vi "Facade.vi"(0 "Data In":T6, 2 "Display State In":T3, 3 "Container State":T5) -> (6 "Data Out":T6, 7 "Display State Out":T3, 8 "Action":T2)   [LabVIEW 2017, in "3D Mesh.xctl"]
uses:
  <vilib>/Math Plots/3D Math Plots/3D Mesh/3D Mesh XCtrl/3D Mesh.xctl
  <vilib>/Math Plots/3D Math Plots/3D Mesh/3D Mesh XCtrl/Data.ctl
  <vilib>/Math Plots/3D Math Plots/3D Plot/3D Plot Datatype/3D Plot Datatype.lvclass
  <vilib>/_xctls/Container State.ctl
  <vilib>/Math Plots/3D Math Plots/3D Mesh/3D Mesh XCtrl/State.ctl
  <vilib>/Math Plots/3D Math Plots/3D Mesh/3D Mesh/3D Mesh.lvclass
  e:/builds/penguin/labview/branches/2017/dev/dist/vi.lib/Math Plots/3D Math Plots/3D Plot/3D Plot/3D Plot.lvclass
  <vilib>/Math Plots/3D Math Plots/3D Plot/Action String/3DMathPlot Ctrl Act Queue.ctl
  <vilib>/Math Plots/3D Math Plots/3D Plot/Action String/3DMathPlot Ctrl Act Cluster.ctl
  <vilib>/Math Plots/3D Math Plots/3D Plot/Action String/3DMathPlot State Class.ctl
  <vilib>/_xctls/Action.ctl
  <vilib>/Math Plots/3D Math Plots/3D Plot/3D Plot/Typedef/Plot Action.ctl
  <vilib>/Math Plots/3D Math Plots/3D Plot/Action String/3DMathPlot Action String.ctl
  <vilib>/_xctls/XControlSupport.lvlib
  <vilib>/Math Plots/3D Math Plots/3D Plot/3D Plot/3D Plot.lvclass
panel:
  out "Export Image":picture
  out "3D Picture Control":refnum<vi>(3d-picture)
  in  "XY Graph":cluster{dbl, dbl}[](graph)
  out "Render Window":refnum<vi>
  in  "Projection Palette":T1
  out "Intensity Graph":dbl[][](graph)
  in  "Color Ramp Palette":cluster{"Active Plot":i32} {"Active Plot" items=["Plot-1"]}
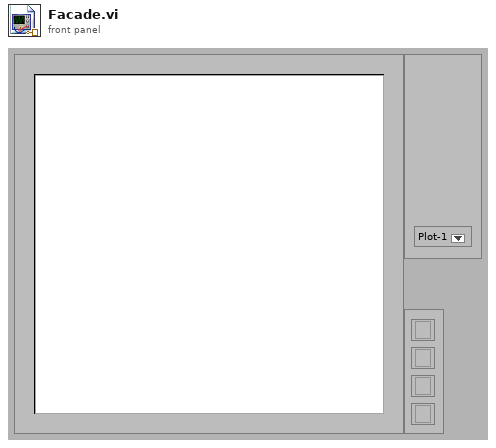
[diagram p1: front panel]
types:
  T1 = cluster{"XY Projection":bool, "XZ Projection":bool, "YZ Projection":bool, "3D Projection":bool}
  T2 = typedef "XControlSupport.lvlib/Action.ctl" = cluster{"Data Changed?":bool, "State Changed?":bool, "Action Name":string}
  T3 = typedef "3D Mesh.xctl/State.ctl" = cluster{"3D Mesh.lvclass":refnum<class "3D Mesh.lvclass">, "Control Ref Queue":T4, "Main Frame Color":u32, "Ramp Palette Color":u32, "Projection Palette Color":u32}
  T4 = typedef "3DMathPlot Ctrl Act Queue.ctl" = refnum<queue>
  T5 = typedef "XControlSupport.lvlib/Container State.ctl" = cluster{"Indicator?":bool, "Run Mode?":bool, " Refnum":refnum<vi>}
  T6 = typedef "3D Mesh.xctl/Data.ctl" = refnum<class "3D Plot Datatype.lvclass">[]
  T7 = typedef "3DMathPlot Ctrl Act Cluster.ctl" = cluster{"3D Picture Control":refnum<vi>, "Render Window Refnum":refnum<vi>, "XY Graph":refnum<vi>, "Intensity Graph":refnum<vi>, "Color Legend Palette":refnum<vi>, "Projection Palette":refnum<vi>, "XControl  Ref":refnum<vi>, "Facade Ref":refnum<vi>, "Export Image Ref":refnum<vi>, "Clear Data Flag":bool, "Display State Change Class":T8}
  T8 = typedef "3DMathPlot State Class.ctl" = enum16{"Update All Objects (Undo)", "Update Light Object Only", "Update Axis Object Only", "Update Plot Object Only", "Update Cursor Object Only", "Update Axis Plot Cursor Objects", "No Update"}
  T9 = typedef "3D Plot.lvclass/Plot Action.ctl" = cluster{"Light Action":enum16{"Update", "Remove", "Nothing"}, "Axis Action":enum16{"Update", "Remove", "Nothing"}, "Plot Action":enum16{"Update", "Remove", "Nothing"}, "Cursor Action":enum16{"Update", "Remove", "Nothing"}, "Fast Draw Action":enum16{"Update", "Remove", "Nothing"}}
  T10 = enum32{"Towards X-Y Plane", "Towards X-Z Plane", "Towards Y-Z Plane", "User Defined"}
  T11 = typedef "3D Plot.lvclass/Actual Transform.ctl" = cluster{"Scale Cluster":cluster{"X Scale":sgl, "Y Scale":sgl, "Z Scale":sgl}, "Translate Cluster":cluster{"X Translate":sgl, "Y Translate":sgl, "Z Translate":sgl}, "Actual Range":T12}
  T12 = typedef "3D Plot.lvclass/Range Clusters.ctl" = cluster{"X Range":cluster{"Max X":sgl, "Min X":sgl}, "Y Range":cluster{"Max Y":sgl, "Min Y":sgl}, "Z Range":cluster{"Max Z":sgl, "Min Z":sgl}}
  T13 = typedef "3D Plot.lvclass/Multiplot Representation.ctl" = cluster{"Plot Represention Array":T14[], "Max Range":T12}
  T14 = typedef "3D Plot.lvclass/Plot Representation.ctl" = cluster{"Plot ID":i32, "Plot Range":T12, "Mesh Data":T15, "Dimension":cluster{"X Dimension":i32, "Y Dimension":i32}, "Ramp Range":T12}
  T15 = typedef "3D Plot.lvclass/Mesh Data.ctl" = cluster{"Index Array":u32[], "Vertex Array":cluster{"X":sgl, "Y":sgl, "Z":sgl}[], "Normal Array":cluster{"X":sgl, "Y":sgl, "Z":sgl}[], "Color Index Array":i32[]}
  T16 = typedef "3D Plot.lvclass/Object Cluster.ctl" = cluster{"Root Scene Object":refnum<vi>, "Fast Root Scene Object":refnum<vi>}
  T17 = typedef "3DMathPlot Action String.ctl" = u16
  T18 = typedef "3D Plot.lvclass/Property Cluster.ctl" = cluster{"Graph Property":T19, "Light Property":T23, "Axis Property":T25, "Value Pair Property":T31, "Format Property":T33, "Cursor Property Array":T34, "Appearance Property":T43}
  T19 = typedef "3D Plot.lvclass/Graph Property.ctl" = cluster{"General Property":T20, "View Property":T21, "Grid Plane":T22}
  T20 = typedef "3D Plot.lvclass/General Property.ctl" = cluster{"Plot Area Color":u32, "Fast Draw?":bool, "Clip Data?":bool}
  T21 = typedef "3D Plot.lvclass/View Property.ctl" = cluster{"Projection Mode":enum16{"Orthographic", "Perspective"}, "View Direction":enum32{"Towards X-Y Plane", "Towards X-Z Plane", "Towards Y-Z Plane", "User Defined"}, "User Defined View Direction":cluster{"View Latitude":sgl, "View Longitude":sgl, "View Distance":sgl}}
  T22 = typedef "3D Plot.lvclass/Grid Plane.ctl" = cluster{"Grid Plane Visible":cluster{"Draw Grid Plane X-Y":bool, "Draw Grid Plane Y-Z":bool, "Draw Grid Plane X-Z":bool}, "Grid Antialiasing":bool, "Grid Frame Color":u32}
  T23 = typedef "3D Plot.lvclass/Light Property.ctl" = cluster{"Enable Lighting?":bool, "Ambient Color":u32, "Light Array":T24[]}
  T24 = typedef "3D Plot.lvclass/Light Specific.ctl" = cluster{"Enable Light?":bool, "Light Color":u32, "Light Latitude":sgl, "Light Longitude":sgl, "Light Distance":sgl, "Attenuation":enum16{"None", "Linear", "Quadratic"}}
  T25 = typedef "3D Plot.lvclass/Axis Property.ctl" = cluster{"Caption Property":T26, "Label Property":T27, "Range Property":T28, "Grid Property":T29, "Ticks Property":T30}
  T26 = typedef "3D Plot.lvclass/Caption Property.ctl" = cluster{"Show Caption":cluster{"Show Normal X Caption":bool, "Show Normal Y Caption":bool, "Show Normal Z Caption":bool, "Show Opposite X Caption":bool, "Show Opposite Y Caption":bool, "Show Opposite Z Caption":bool}, "Caption Color":cluster{"Caption Color X":u32, "Caption Color Y":u32, "Caption Color Z":u32}, "Caption Size":cluster{"Caption Size X":u16, "Caption Size Y":u16, "Caption Size Z":u16}, "Caption String":cluster{"Caption X":string, "Caption Y":string, "Caption Z ":string}}
  T27 = typedef "3D Plot.lvclass/Label Property.ctl" = cluster{"Show Label":cluster{"Show Normal X Label":bool, "Show Normal Y Label":bool, "Show Normal Z Label":bool, "Show Opposite X Label":bool, "Show Opposite Y Label":bool, "Show Opposite Z Label":bool}, "Label Color":cluster{"Label Color X":u32, "Label Color Y":u32, "Label Color Z":u32}, "Label Size":cluster{"Label Size X":u16, "Label Size Y":u16, "Labe Size Z":u16}}
  T28 = typedef "3D Plot.lvclass/Range Property.ctl" = cluster{"Range Cluster":T12, "Auto Range":cluster{"Auto Range X":bool, "Auto Range Y":bool, "Auto Range Z":bool}, "Inverted":cluster{"Inverted X":bool, "Inverted Y":bool, "Inverted Z":bool}, "Logarithm":cluster{"Logarithm X":bool, "Logarithm Y":bool, "Logarithm Z":bool}}
  T29 = typedef "3D Plot.lvclass/Grid Property.ctl" = cluster{"Major Grid Visible":cluster{"Draw Major Grid X":bool, "Draw Major Grid Y":bool, "Draw Major Grid Z":bool}, "Major Grid Color":cluster{"Major Grid Color X":u32, "Major Grid Color Y":u32, "Major Grid Color Z":u32}, "Minor Grid Visible":cluster{"Draw Minor Grid X":bool, "Draw Minor Grid Y":bool, "Draw Minor Grid Z":bool}, "Minor Grid Color":cluster{"Minor Grid Color X":u32, "Minor Grid Color Y":u32, "Minor Grid Color Z":u32}}
  T30 = typedef "3D Plot.lvclass/Tick Property.ctl" = cluster{"Major Tick Visible":cluster{"Draw Major Tick X":bool, "Draw Major Tick Y":bool, "Draw Major Tick Z":bool}, "Major Tick Color":cluster{"Major Tick Color X":u32, "Major Tick Color Y":u32, "Major Tick Color Z":u32}, "Major Count":cluster{"Major Count X":u16, "Major Count Y":u16, "Major Count Z":u16}, "Minor Tick Visible":cluster{"Draw Minor Tick X":bool, "Draw Minor Tick Y":bool, "Draw Minor Tick Z":bool}, "Minor Tick Color":cluster{"Minor Tick Color X":u32, "Minor Tick Color Y":u32, "Minor Tick Color Z":u32}, "Minor Count":cluster{"Minor Count X":u16, "Minor Count Y":u16, "Minor Count Z":u16}}
  T31 = typedef "3D Plot.lvclass/Value Pair Property.ctl" = T32[]
  T32 = typedef "3D Plot.lvclass/Value Pair Cluster.ctl" = cluster{"Value Pair Array":cluster{"Value":sgl, "Name":string}[], "Show Tick":bool, "Show Grid":bool, " Label Mode":enum16{"Name", "Value", "None"}}
  T33 = typedef "3D Plot.lvclass/Format Property.ctl" = string[]
  T34 = typedef "3D Plot.lvclass/Cursor Property Array.ctl" = T35[]
  T35 = typedef "3D Plot.lvclass/Cursor Property.ctl" = cluster{"Cursor Visible":bool, "Cursor Enable":bool, "Cursor Position":T36, "Cursor Point":T37, "Cursor Line":T39, "Cursor Plane":T41, "Cursor Text":T42}
  T36 = typedef "3D Plot.lvclass/Cursor Position.ctl" = cluster{"Cursor Plot ID":i32, "Cursor X":sgl, "Cursor Y":sgl, "Cursor Z":sgl, "Cursor Snap To":enum16{"Fixed", "Nearest Plot", "Snap to Plot"}}
  T37 = typedef "3D Plot.lvclass/Cursor Point.ctl" = cluster{"Cursor Point Color":u32, "Cursor Point Size":sgl, "Cursor Point Style":T38}
  T38 = typedef "3D Plot.lvclass/Sprite Type.ctl" = enum16{"None", "Empty Square", "Solid Square", "Empty Diamond", "Solid Diamond", "Empty Circle", "Solid Circle", "Asterisk", "Bold X", "Wireframe Sphere", "Solid Sphere", "Wireframe Cube", "Solid Cube"}
  T39 = typedef "3D Plot.lvclass/Cursor Line.ctl" = cluster{"Cursor Line Color":u32, "Cursor Line Width":sgl, "Cursor Line Style":T40}
  T40 = typedef "3D Plot.lvclass/Line Type.ctl" = enum16{"None", "Solid", "Dash", "Dot", "Dash Dot"}
  T41 = typedef "3D Plot.lvclass/Cursor Plane.ctl" = cluster{"Cursor Plane Color":u32, "Cursor Plane Opacity":sgl, "Draw Cursor Plane X-Z":bool, "Draw Cursor Plane Y-Z":bool, "Draw Cursor Plane X-Y":bool}
  T42 = typedef "3D Plot.lvclass/Cursor Text.ctl" = cluster{"Cursor Text":string, "Cursor Text Size":u16, "Cursor Show Position":bool, "Cursor Show Name":bool, "Cursor Text Color":u32, "Background Color":u32, "Background Opacity":sgl}
  T43 = typedef "3D Plot.lvclass/Apearance Property.ctl" = cluster{"Visibility":T44, "Active Index":cluster{"Active Plot":i32, "Active Cursor":i32, "Active Axis":enum16{"X-axis", "Y-axis", "Z-axis"}, "Active Value Pair":enum16{"X-axis", "Y-axis", "Z-axis"}, "Active Light":enum16{"Light 0", "Light 1", "Light 2", "Light 3"}}, "Backup Data":cluster{"Plot Name":string[]}}
  T44 = typedef "3D Plot.lvclass/Item Visibility.ctl" = cluster{"Projection Palette":bool, "Color Ramp Palette":bool}
  T45 = typedef "LVPoint32TypeDef.ctl" = cluster{"Horizontal":i32, "Vertical":i32}
  T46 = typedef "LVRangeTypeDef.ctl" = cluster{"Minimum":dbl, "Maximum":dbl, "Increment":dbl, "Minor Increment":dbl, "Start":dbl}
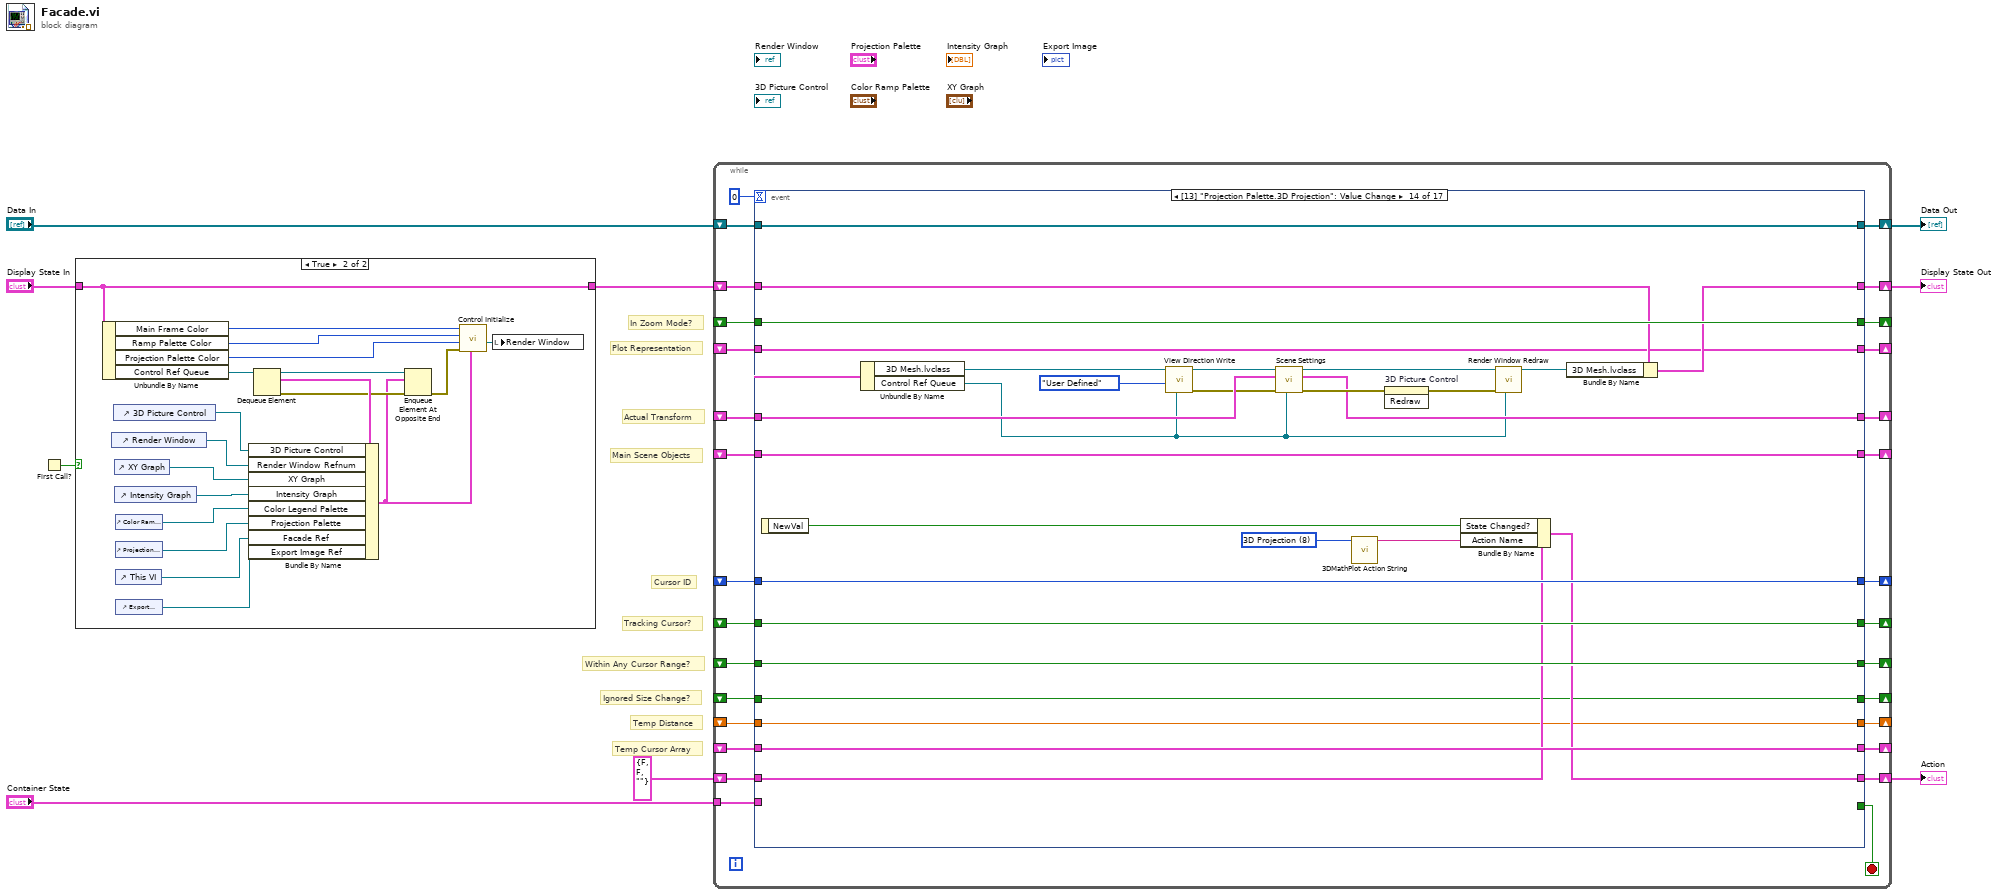
[diagram p0: block diagram]
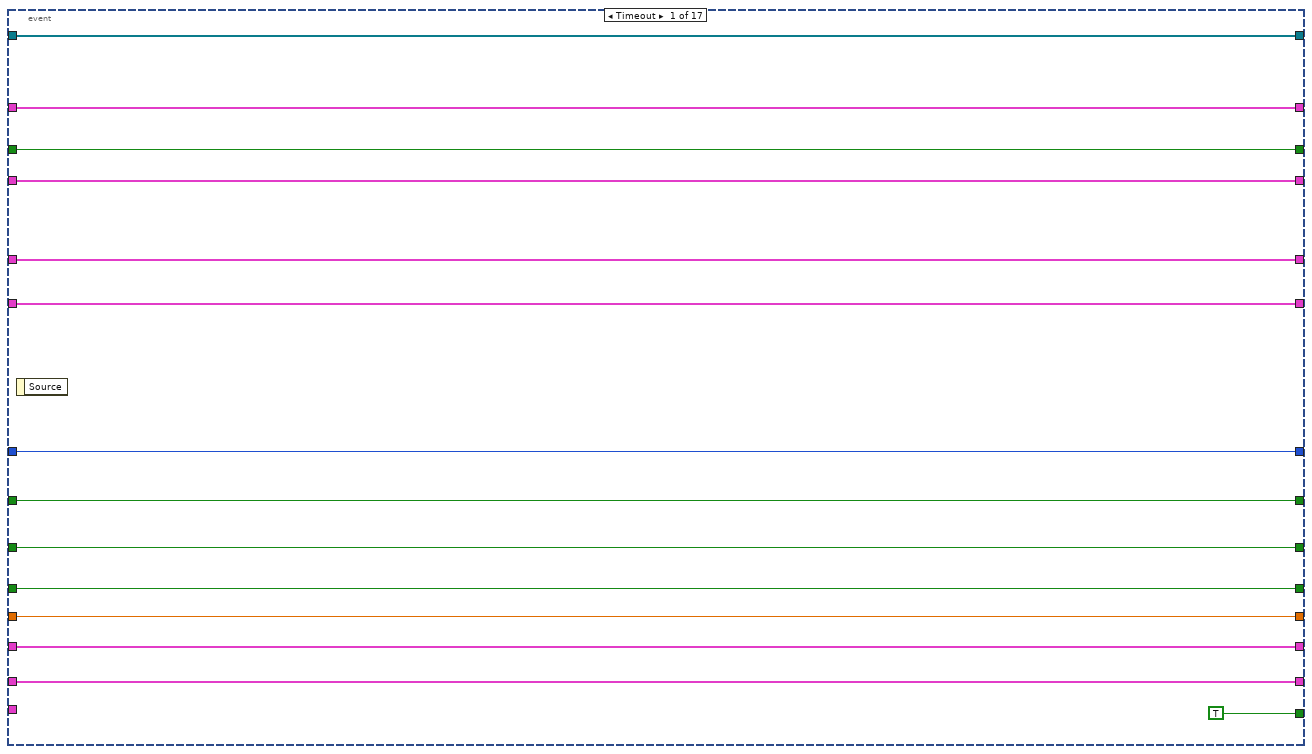
[diagram p3: hidden frame]
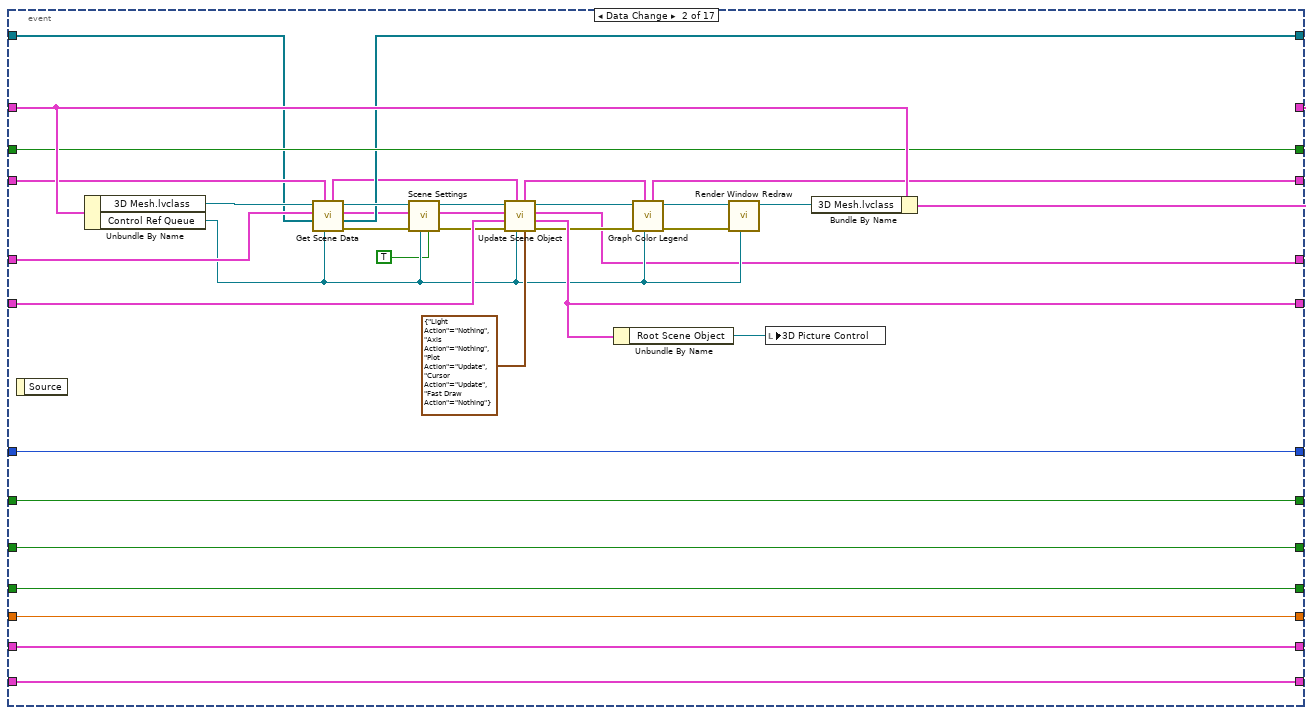
[diagram p4: hidden frame]
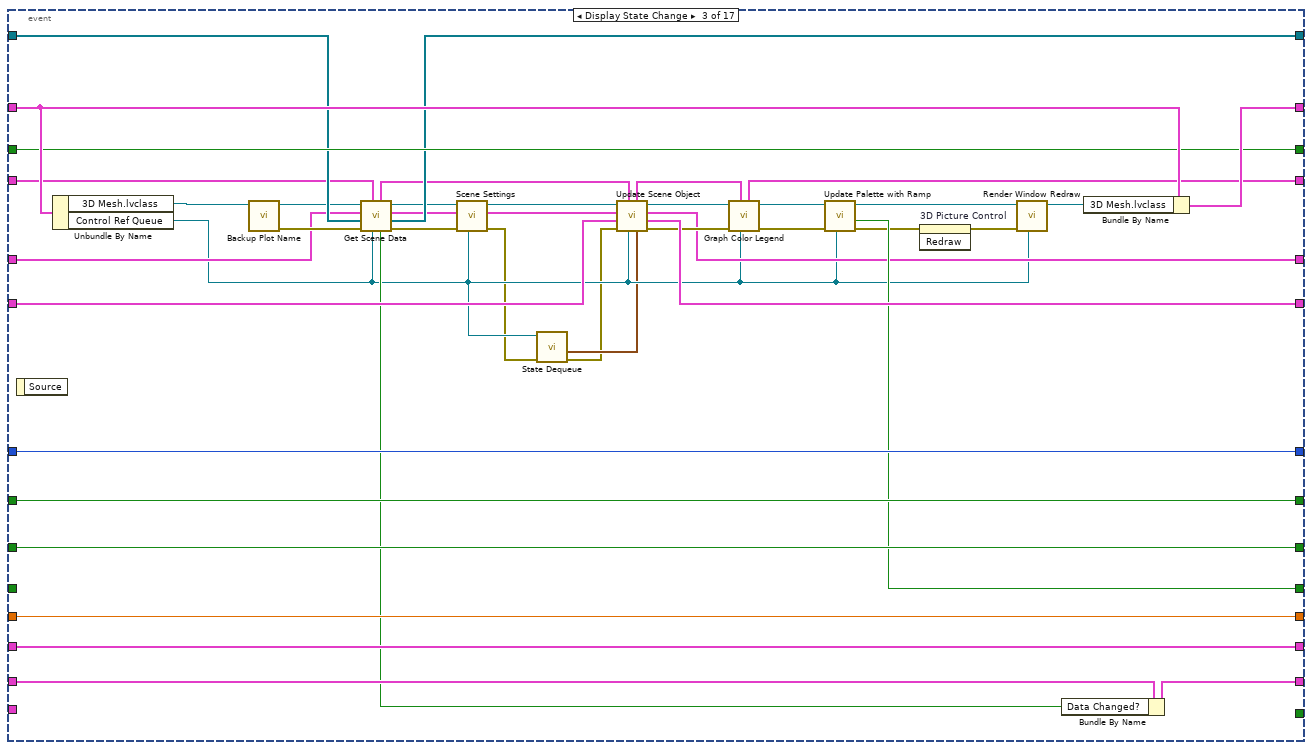
[diagram p5: hidden frame]
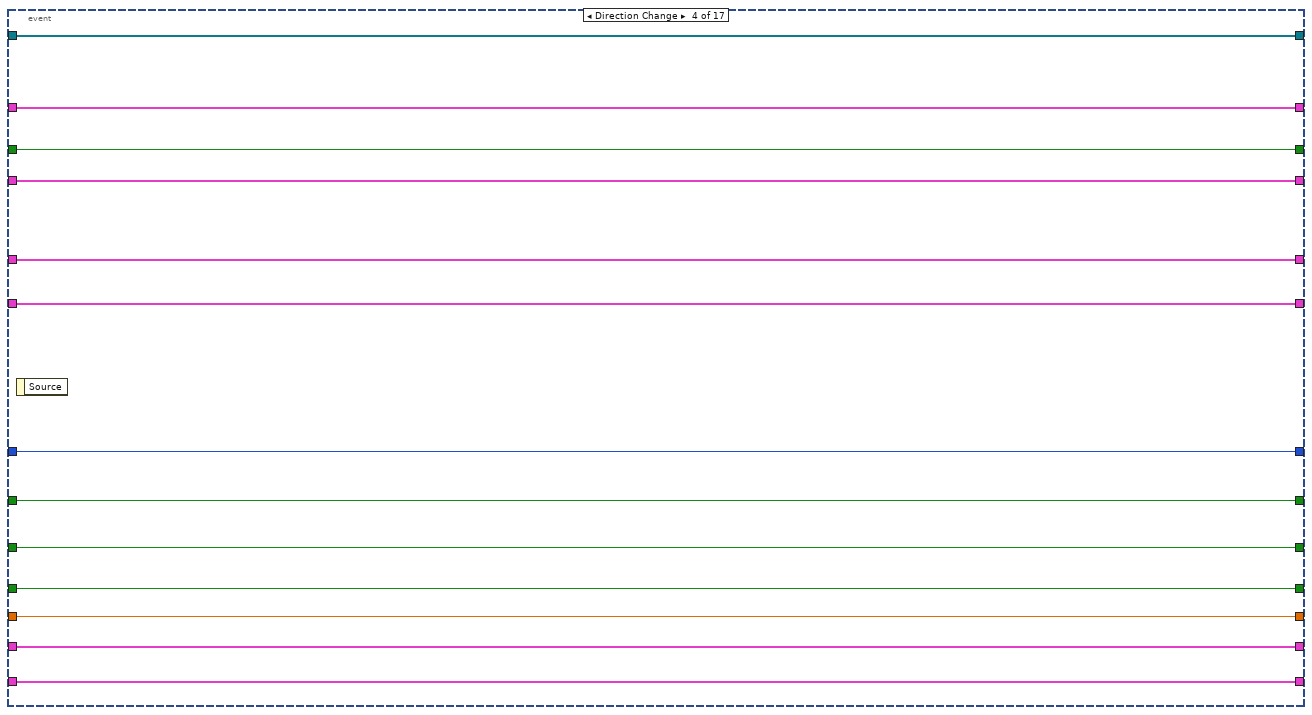
[diagram p6: hidden frame]
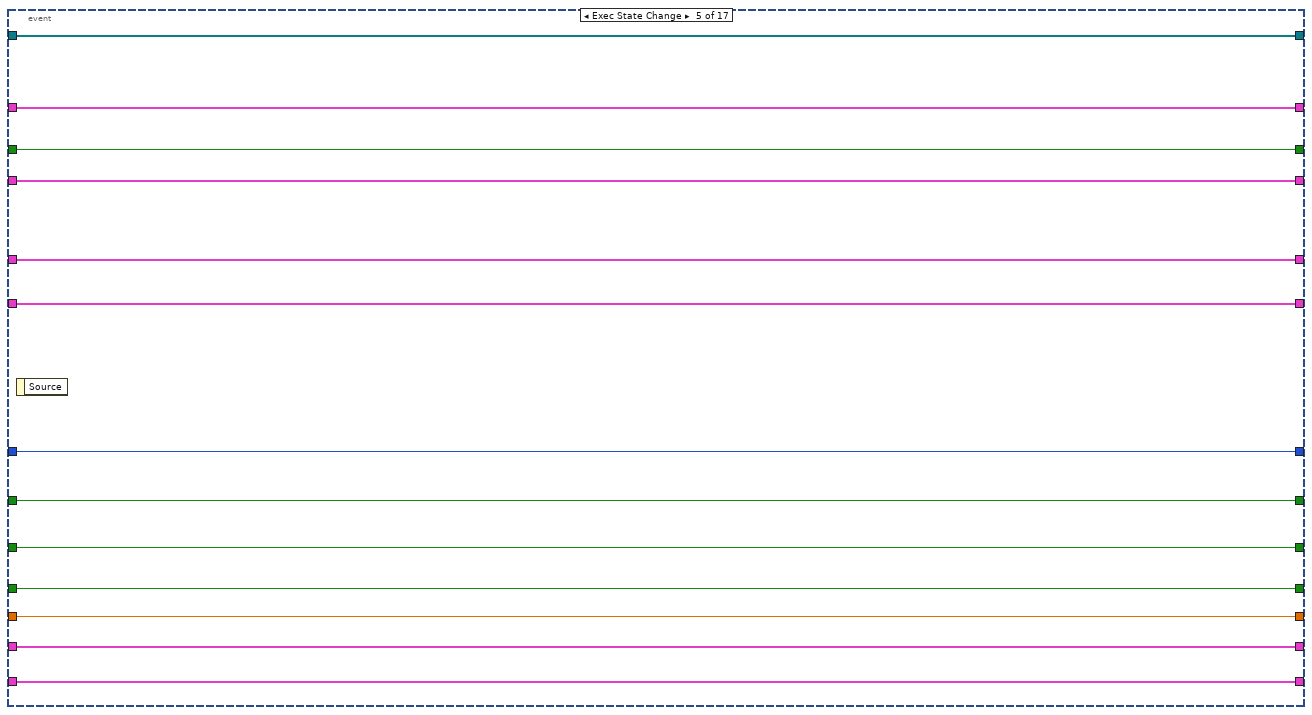
[diagram p7: hidden frame]
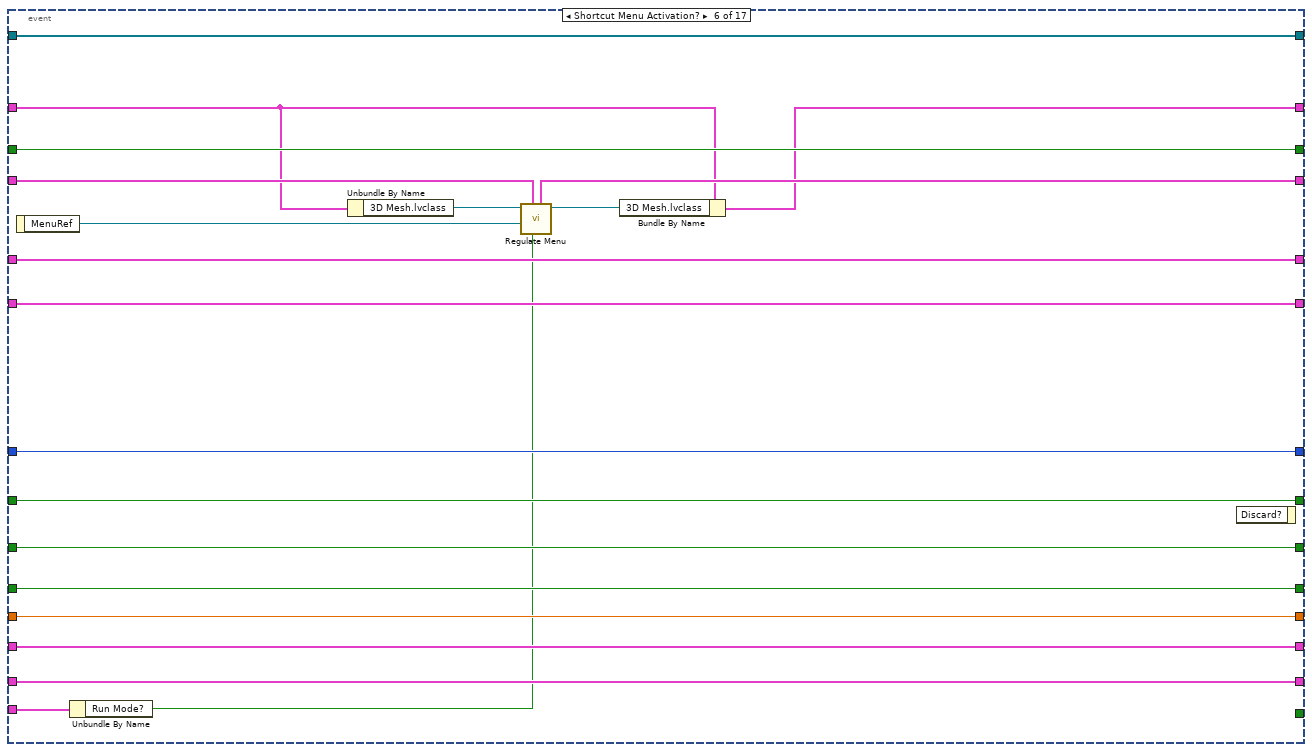
[diagram p8: hidden frame]
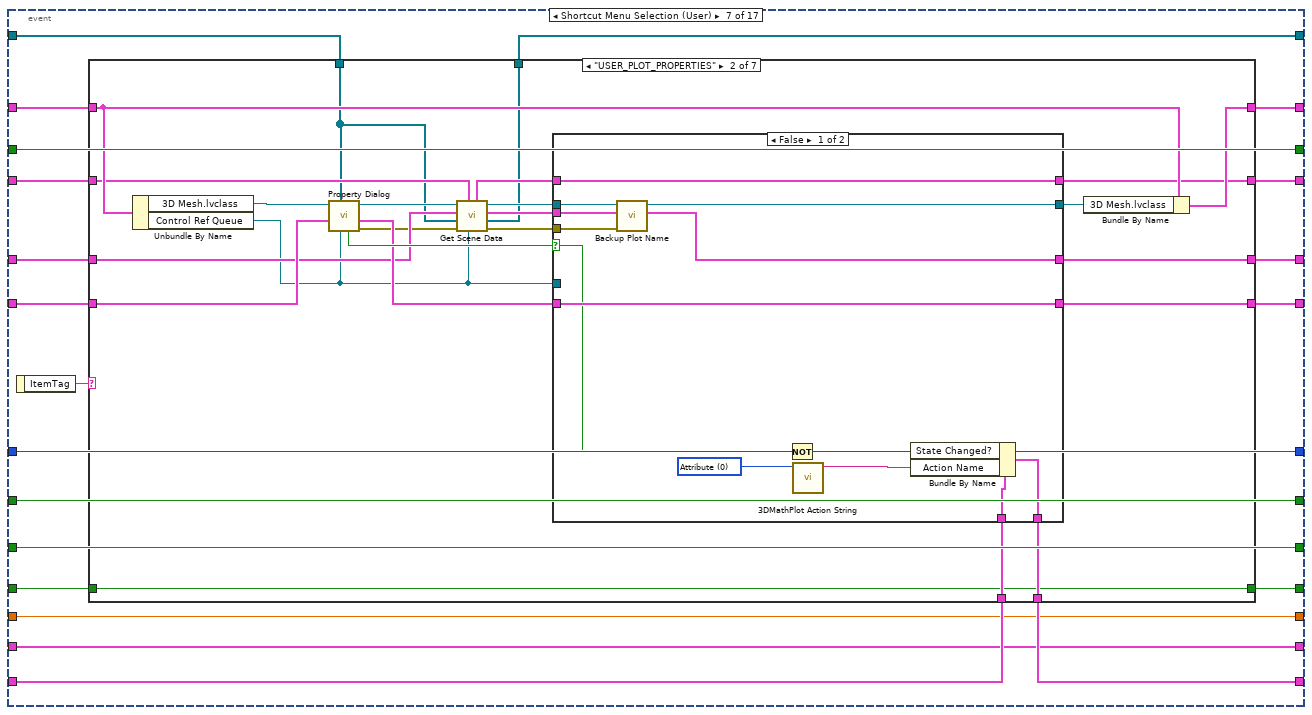
[diagram p9: hidden frame]
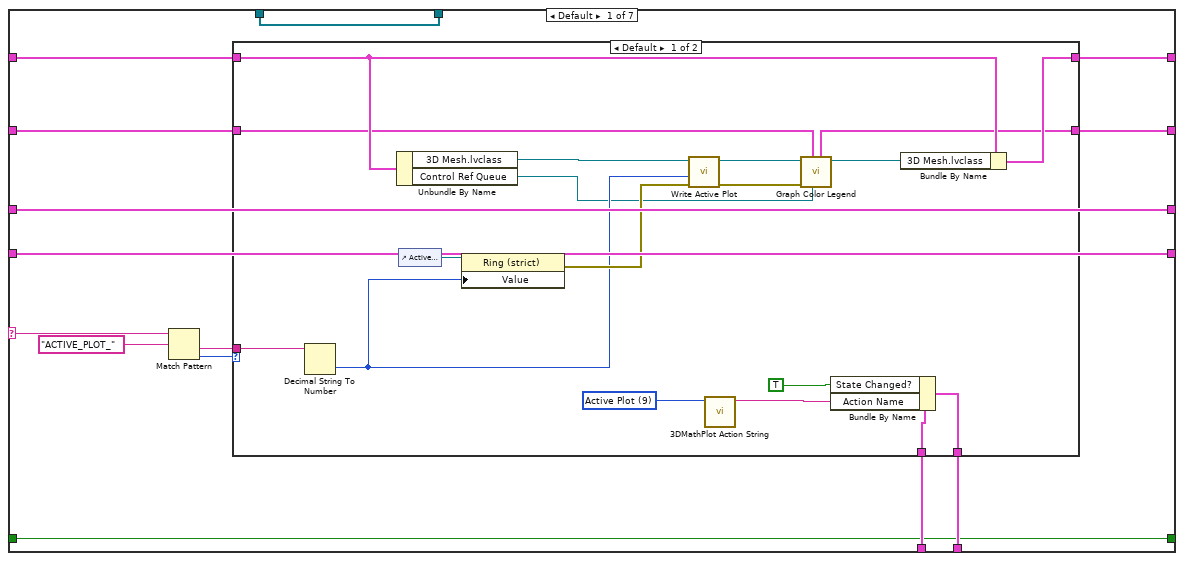
[diagram p10: hidden frame]
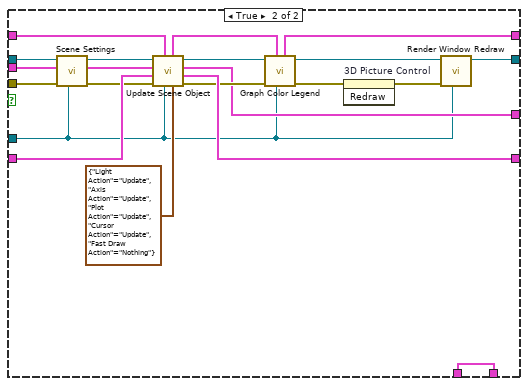
[diagram p12: hidden frame]
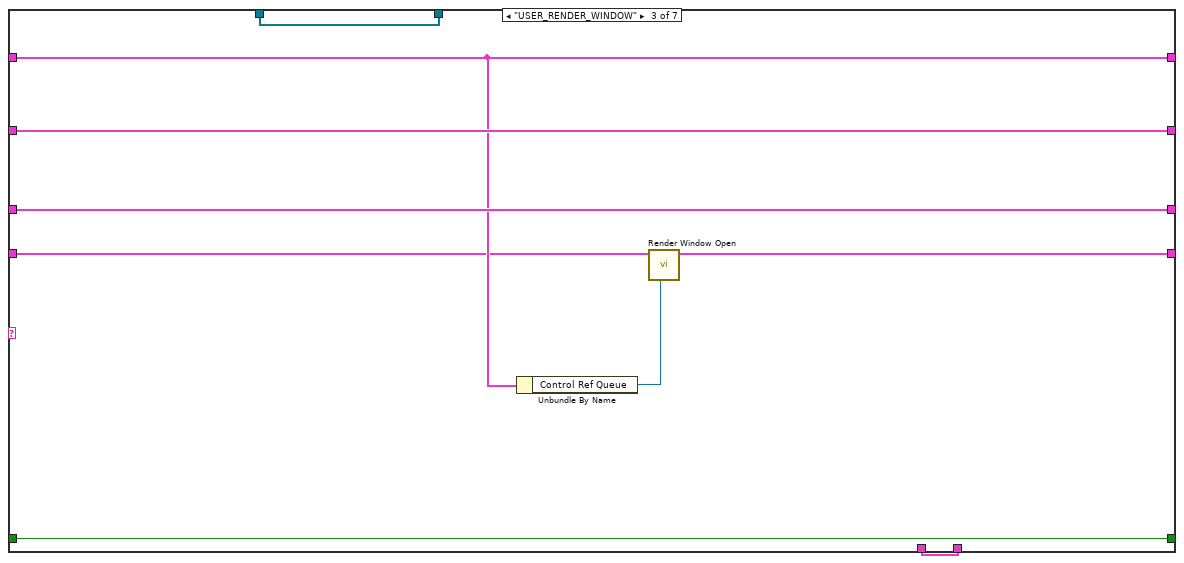
[diagram p13: hidden frame]
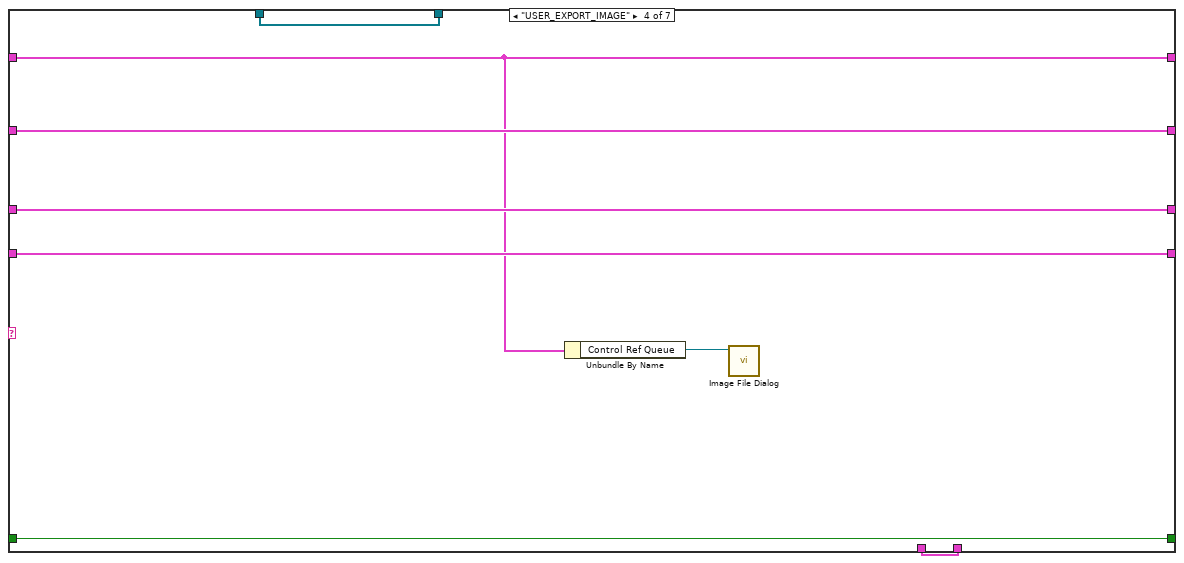
[diagram p14: hidden frame]
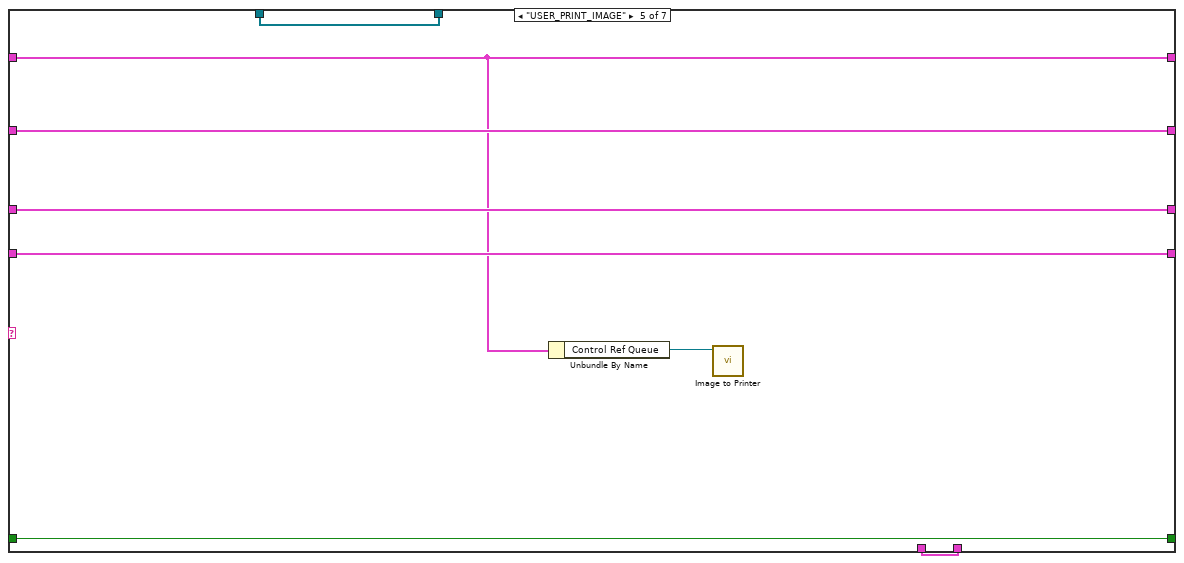
[diagram p15: hidden frame]
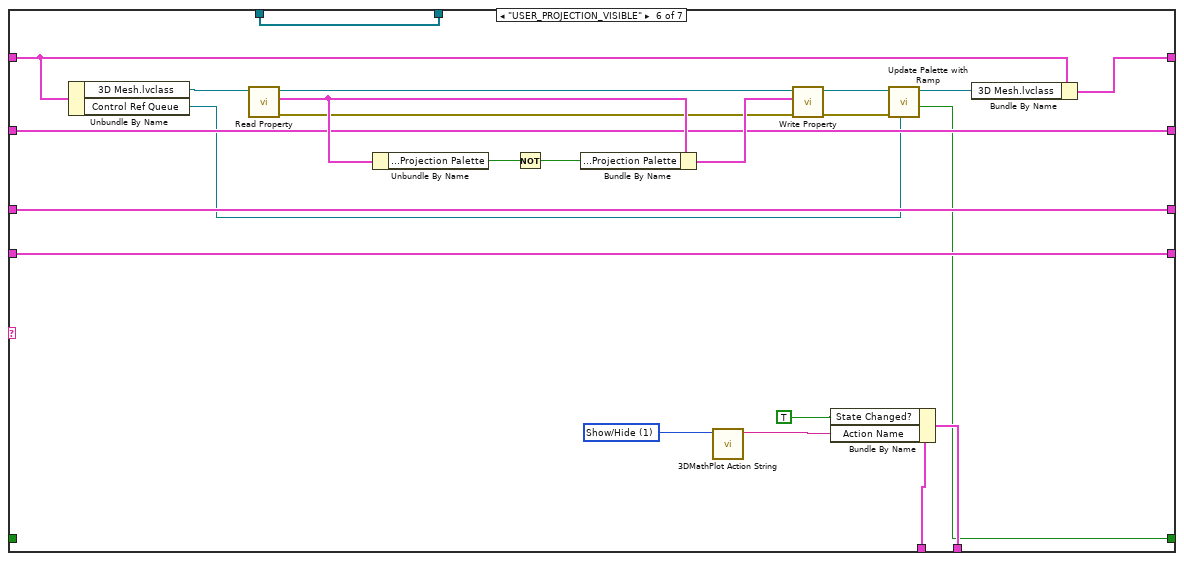
[diagram p16: hidden frame]
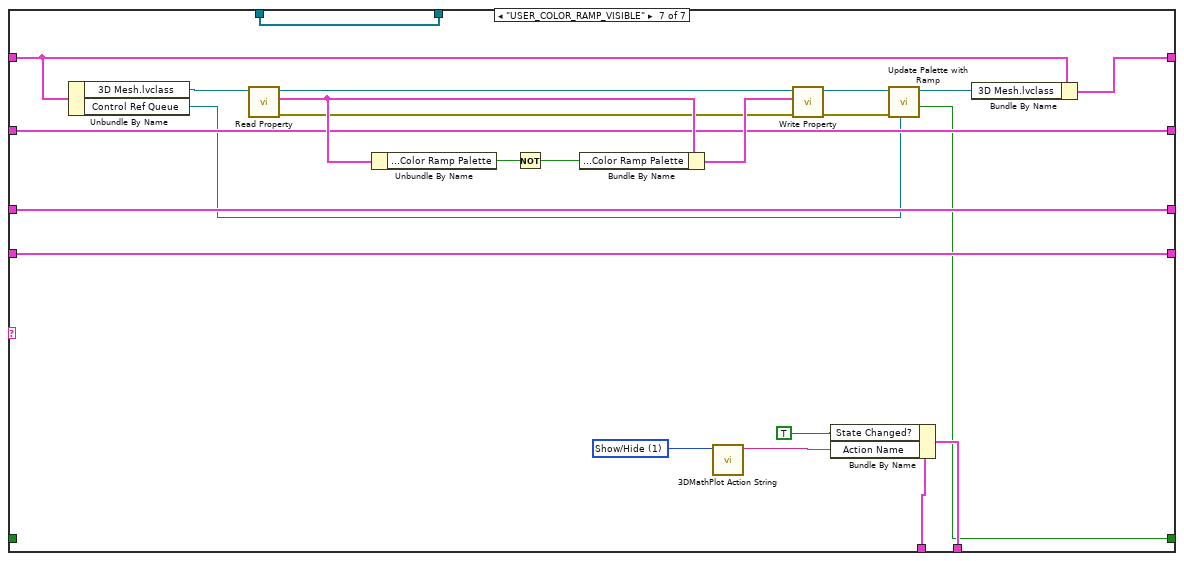
[diagram p17: hidden frame]
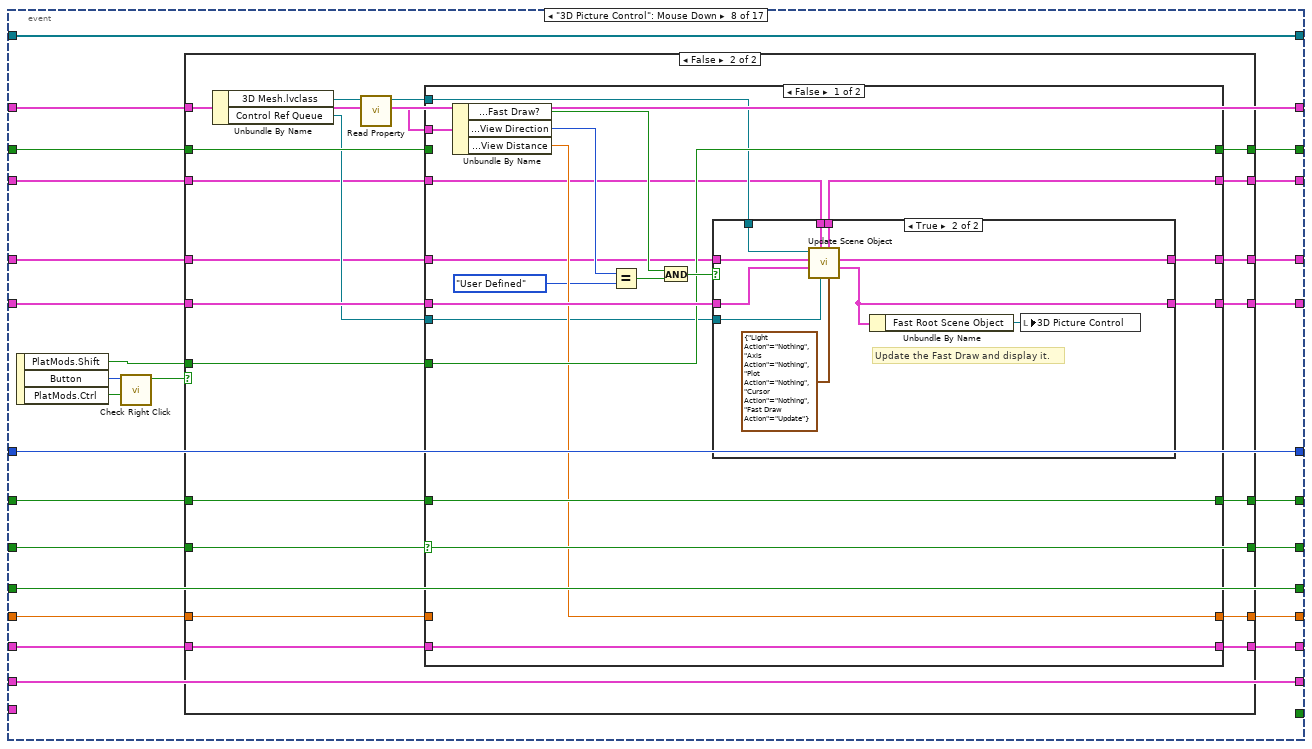
[diagram p18: hidden frame]
diagram:
  # "Ignored Size Change?"
  # "Actual Transform"
  # "Temp Cursor Array"
  # "Temp Distance"
  # "Within Any Cursor Range?"
  # "Tracking Cursor?"
  # "Cursor ID"
  # "Plot Representation"
  # "In Zoom Mode?"
  # "Main Scene Objects"
  n1 = First Call?() -> (First Call?: T/F=w4:bool)
  n2 = case shown="True" w4 {
    tunnel: [w10 w15] -> w3
    tunnel: "Display State In" -> [w10 w15]
    frame False {
    }
    frame True {
      n3 = Unbundle By Name(w15) -> ("Main Frame Color"=w13:u32, "Ramp Palette Color"=w12:u32, "Projection Palette Color"=w11:u32, "Control Ref Queue"=w16:T4)
      n4 = control-ref of="Render Window"() -> (w27:refnum<vi>)
      n5 = control-ref of="3D Picture Control"() -> (w28:refnum<vi>)
      n6 = control-ref of="XY Graph"() -> (w22:refnum<vi>)
      n7 = control-ref of="Intensity Graph"() -> (w26:refnum<vi>)
      n8 = control-ref of="Color Ramp Palette"() -> (w25:refnum<vi>)
      n9 = control-ref of="Projection Palette"() -> (w24:refnum<vi>)
      n10 = control-ref of="This VI"() -> (w23:refnum<vi>)
      n11 = control-ref of="Export Image"() -> (w14:refnum<vi>)
      n12 = Dequeue Element(queue=w16) -> (queue out=w20:T4, element=w21:T7, error out=w19:errorcluster)  [unwired: 1 in, 2 out]
      n13 = Bundle By Name(cluster=w21, "3D Picture Control"=w28, "Render Window Refnum"=w27, "XY Graph"=w22, "Intensity Graph"=w26, "Color Legend Palette"=w25, "Projection Palette"=w24, "Facade Ref"=w23, "Export Image Ref"=w14) -> (w17:T7)
      n14 = Enqueue Element At Opposite End(queue=w20, element=w17, error in (no error)=w19) -> (error out=w18:errorcluster)  [unwired: 3 out]
      n15 = call <vilib>:"Control Initialize.vi"("Control Ref Cluster"=w17, "error in (no error)"=w18, "Projection Palette Color"=w11, "Ramp Palette Color"=w12, "Main Frame Color"=w13) -> ("New Window Refnum"=w29:refnum<vi>)  [unwired: 6 out]
      n16 = local write "Render Window"(w29) -> ()
    }
  }
  n17 = while {
    shift-right: [w57] -> w7
    shift-left: w3 -> [w58]
    tunnel: "Container State" -> [w54]
    shift-right: [w53] -> w9
    shift-left: "Data In" -> [w48]
    shift-right: [w51] -> w6
    shift-left: T2 {"Data Changed?"=FALSE, "State Changed?"=FALSE, "Action Name"=""} ("Action") -> [w52]
    shift-right: [w50] -> _
    shift-left: _ -> [w49]
    shift-right: [w47] -> _
    shift-left: _ -> [w34]
    shift-right: [w45] -> _
    shift-left: _ -> [w46]
    shift-right: [w44] -> _
    shift-left: _ -> [w43]
    shift-right: [w41] -> _
    shift-left: _ -> [w42]
    shift-right: [w40] -> _
    shift-left: _ -> [w39]
    shift-right: [w38] -> _
    shift-left: _ -> [w37]
    shift-right: [w36] -> _
    shift-left: _ -> [w35]
    shift-right: [w33] -> _
    shift-left: _ -> [w32]
    shift-right: [w31] -> _
    shift-left: _ -> [w30]
    stop <- w56 stop-if-true
    n18 = event shown="[13] \"Projection Palette.3D Projection\": Value Change" {
      selector: _ -> [_ _ _ _ _ _ _ _ _ _ _ _ _ _ _ _ _]
      dyn-events: _ -> [_ _ _ _ _ _ _ _ _ _ _ _ _ _ _ _ _]
      timeout: 0 -> [_ _ _ _ _ _ _ _ _ _ _ _ _ _ _ _ _]
      tunnel: w58 -> [w60 w107 w147 w161 w174 w176 w211 w398 w486 w569 w595 w622 w649 w676 w700 w731 w747]
      tunnel: [w60 w106 w146 w161 w174 w175 w210 w398 w483 w569 w592 w621 w648 w675 w699 w730 w746] -> w57
      tunnel: [TRUE _ _ _ _ _ _ _ _ _ _ _ _ _ _ _ _] -> w56
      tunnel: w54 -> [_ _ _ _ _ w184 _ _ _ _ _ _ _ _ _ _ _]
      tunnel: w48 -> [w70 w82 w137 w160 w173 w194 w199 w402 w489 w573 w601 w628 w655 w682 w707 w740 w755]
      tunnel: [w70 w81 w138 w160 w173 w194 w198 w402 w489 w573 w601 w628 w655 w682 w707 w740 w755] -> w53
      tunnel: [w71 w97 w126 w159 w172 w192 w212 w401 w484 w572 w593 w619 w646 w673 w693 w727 w753] -> w51
      tunnel: w52 -> [w71 w97 w148 w159 w172 w192 w213 w401 w485 w572 w594 w620 w647 w674 w694 w728 w753]
      tunnel: [w62 w96 w140 w158 w171 w193 w214 w381 w487 w566 w585 w613 w639 w667 w688 w726 w754] -> w50
      tunnel: w49 -> [w62 w99 w141 w158 w171 w193 w215 w399 w488 w567 w585 w613 w639 w667 w688 w725 w754]
      tunnel: [w69 w104 w139 w157 w170 w191 w204 w397 w477 w570 w596 w627 w654 w681 w706 w735 w750] -> w47
      tunnel: w34 -> [w69 w104 w139 w157 w170 w191 w204 w396 w481 w571 w596 w627 w654 w681 w706 w735 w750]
      tunnel: w46 -> [w68 w103 w145 w156 w169 w190 w205 w395 w478 w565 w597 w626 w653 w680 w705 w736 w751]
      tunnel: [w68 w103 w145 w156 w169 w190 w205 w395 w478 w564 w597 w626 w653 w680 w705 w736 w751] -> w45
      tunnel: w43 -> [w67 w102 w144 w155 w168 w189 w206 w394 w480 w561 w598 w625 w652 w679 w704 w737 w752]
      tunnel: [w67 w102 w144 w155 w168 w189 w206 w393 w477 w561 w598 w625 w652 w679 w704 w737 w752] -> w44
      tunnel: w42 -> [w66 w101 w143 w154 w167 w188 w207 w392 _ _ w599 w624 w651 w678 w703 w738 w748]
      tunnel: [w66 w101 w143 w154 w167 w188 w207 w391 w477 w560 w599 w624 w651 w678 w703 w738 w748] -> w41
      tunnel: [w65 w100 w142 w153 w166 w187 w208 w390 w479 w563 w600 w623 w650 w677 w702 w739 w749] -> w40
      tunnel: w39 -> [w65 w100 w142 w153 w166 w187 w208 w389 w479 _ w600 w623 w650 w677 w702 w739 w749]
      tunnel: [w63 w75 w113 w152 w165 w178 w202 w383 w475 w559 w577 w610 w637 w664 w683 w713 w742] -> w38
      tunnel: w37 -> [w63 w84 w119 w152 w165 w179 w203 w384 w476 w559 w577 w610 w637 w664 w684 w709 w742]
      tunnel: w35 -> [w64 w83 w120 w151 w164 w186 w201 w385 w474 w558 w579 w609 w636 w663 w689 w712 w743]
      tunnel: [w64 w74 w114 w151 w164 w186 w200 w382 w473 w558 w578 w608 w635 w662 w689 w714 w743] -> w36
      tunnel: [w61 w93 w133 w150 w163 w185 w197 w388 w472 w557 w589 w616 w643 w670 w691 w722 FALSE] -> w33
      tunnel: w32 -> [w61 w93 _ w150 w163 w185 w196 w388 w472 w557 w589 w616 w643 w670 w691 w722 w745]
      tunnel: [w59 w87 w127 w149 w162 w183 w195 w387 w471 w551 w587 w614 w641 w668 w687 w715 w741] -> w31
      tunnel: w30 -> [w59 w87 w127 w149 w162 w183 w195 w386 w471 _ w587 w614 w641 w668 w687 w715 w741]
      event Timeout {
        n19 = event-data() -> ()  [unwired: 2 out]
      }
      event Data Change {
        n20 = event-data() -> ()  [unwired: 2 out]
        n21 = Unbundle By Name(w107) -> ("3D Mesh.lvclass"=w86:refnum<class "3D Mesh.lvclass">, "Control Ref Queue"=w78:T4)
        n22 = call <vilib>:"Get Scene Data.vi"("Control Ref Queue"=w78, "Multiplot Representation In"=w84, "Data In"=w82, "Actual Transform In"=w83, "3D Plot.lvclass in"=w86) -> ("error out"=w79:errorcluster, "Data Out"=w81:refnum<class "3D Plot Datatype.lvclass">[], "Actual Transform Out"=w80:T11, "3D Plot.lvclass out"=w85:refnum<class "3D Mesh.lvclass">, "Multiplot Representation Out"=w77:T13)  [unwired: 1 in, 1 out]
        n23 = call <vilib>:"Scene Settings.vi"("Data Change Event?"=TRUE, "Control Ref Queue"=w78, "error in (no error)"=w79, "Actual Transform In"=w80, "3D Plot.lvclass in"=w85) -> ("error out"=w88:errorcluster, "Actual Transform Out"=w98:T11, "3D Plot.lvclass out"=w89:refnum<class "3D Mesh.lvclass">)  [unwired: 2 in, 2 out]
        n24 = call <vilib>:"Update Scene Object.vi"("Action"=T9 {"Light Action"=enum."Nothing", "Axis Action"=enum."Nothing", "Plot Action"=enum."Update", "Cursor Action"=enum."Update", "Fast Draw Action"=enum."Nothing"}, "Control Ref Queue"=w78, "Multiplot Representation In"=w77, "error in (no error)"=w88, "Object Cluster In"=w99, "Actual Transform In"=w98, "3D Plot.lvclass in"=w89) -> ("error out"=w94:errorcluster, "Object Cluster Out"=w96:T16, "Actual Transform Out"=w74:T11, "3D Plot.lvclass out"=w95:refnum<class "3D Mesh.lvclass">, "Multiplot Representation Out"=w76:T13)
        n25 = Unbundle By Name(w96) -> ("Root Scene Object"=w105:refnum<vi>)
        n26 = call-dynamic "Graph Color Legend.vi"("Control Ref Queue"=w78, "Multiplot Representation In"=w76, "error in (no error)"=w94, "3D Plot.lvclass in"=w95) -> ("error out"=w90:errorcluster, "3D Plot.lvclass out"=w91:refnum<class "3D Mesh.lvclass">, "Multiplot Representation Out"=w75:T13)  [unwired: 2 in, 3 out]
        n27 = call <vilib>:"Render Window Redraw.vi"("Control Ref Queue"=w78, "error in (no error)"=w90) -> ()  [unwired: 1 in, 9 out]
        n28 = local write "3D Picture Control"(w105) -> ()
        n29 = Bundle By Name(cluster=w107, "3D Mesh.lvclass"=w91) -> (w106:T3)
      }
      event Display State Change {
        n30 = event-data() -> ()  [unwired: 2 out]
        n31 = Unbundle By Name(w147) -> ("3D Mesh.lvclass"=w112:refnum<class "3D Mesh.lvclass">, "Control Ref Queue"=w111:T4)
        n32 = call-dynamic "Backup Plot Name.vi"("3D Mesh.lvclass in"=w112) -> ("error out"=w121:errorcluster, "3D Mesh.lvclass out"=w124:refnum<class "3D Mesh.lvclass">)  [unwired: 1 in, 8 out]
        n33 = call <vilib>:"Get Scene Data.vi"("Control Ref Queue"=w111, "Multiplot Representation In"=w119, "error in (no error)"=w121, "Data In"=w137, "Actual Transform In"=w120, "3D Plot.lvclass in"=w124) -> ("error out"=w123:errorcluster, "Data Out"=w138:refnum<class "3D Plot Datatype.lvclass">[], "Actual Transform Out"=w118:T11, "3D Plot.lvclass out"=w122:refnum<class "3D Mesh.lvclass">, "Data Cleaned?"=w125:bool, "Multiplot Representation Out"=w116:T13)
        n34 = call <vilib>:"Scene Settings.vi"("Control Ref Queue"=w111, "error in (no error)"=w123, "Actual Transform In"=w118, "3D Plot.lvclass in"=w122) -> ("error out"=w108:errorcluster, "Actual Transform Out"=w117:T11, "3D Plot.lvclass out"=w128:refnum<class "3D Mesh.lvclass">)  [unwired: 3 in, 2 out]
        n35 = call <vilib>:"State Dequeue.vi"("error in (no error)"=w108, "Control Ref Queue"=w111) -> ("error out"=w109:errorcluster, "Action"=w110:T9)  [unwired: 8 out]
        n36 = call <vilib>:"Update Scene Object.vi"("Action"=w110, "Control Ref Queue"=w111, "Multiplot Representation In"=w116, "error in (no error)"=w109, "Object Cluster In"=w141, "Actual Transform In"=w117, "3D Plot.lvclass in"=w128) -> ("error out"=w135:errorcluster, "Object Cluster Out"=w140:T16, "Actual Transform Out"=w114:T11, "3D Plot.lvclass out"=w136:refnum<class "3D Mesh.lvclass">, "Multiplot Representation Out"=w115:T13)
        n37 = call-dynamic "Graph Color Legend.vi"("Control Ref Queue"=w111, "Multiplot Representation In"=w115, "error in (no error)"=w135, "3D Plot.lvclass in"=w136) -> ("error out"=w131:errorcluster, "3D Plot.lvclass out"=w132:refnum<class "3D Mesh.lvclass">, "Multiplot Representation Out"=w113:T13)  [unwired: 2 in, 3 out]
        n38 = call <vilib>:"Update Palette with Ramp.vi"("Control Ref Queue"=w111, "error in (no error)"=w131, "3D Plot.lvclass in"=w132) -> ("error out"=w130:errorcluster, "Ignore the size change?"=w133:bool, "3D Plot.lvclass out"=w134:refnum<class "3D Mesh.lvclass">)  [unwired: 6 out]
        n39 = invoke on="3D Picture Control" class="SceneGraphDisp (strict)" method="Redraw"(error in=w130) -> (error out=w129:errorcluster)  [unwired: 2 in, 2 out]
        n40 = call <vilib>:"Render Window Redraw.vi"("Control Ref Queue"=w111, "error in (no error)"=w129) -> ()  [unwired: 1 in, 9 out]
        n41 = Bundle By Name(cluster=w148, "Data Changed?"=w125) -> (w126:T2)
        n42 = Bundle By Name(cluster=w147, "3D Mesh.lvclass"=w134) -> (w146:T3)
      }
      event Direction Change {
        n43 = event-data() -> ()  [unwired: 2 out]
      }
      event Exec State Change {
        n44 = event-data() -> ()  [unwired: 2 out]
      }
      event Shortcut Menu Activation? {
        n45 = event-data() -> ("MenuRef"=w181:refnum<k9>)  [unwired: 1 out]
        n46 = Unbundle By Name(w184) -> ("Run Mode?"=w180:bool)
        n47 = Unbundle By Name(w176) -> ("3D Mesh.lvclass"=w182:refnum<class "3D Mesh.lvclass">)
        n48 = call <vilib>:"Regulate Menu.vi"("Run Mode?"=w180, "Multiplot Representation In"=w179, "MenuRef"=w181, "3D Plot.lvclass in"=w182) -> ("3D Plot.lvclass out"=w177:refnum<class "3D Mesh.lvclass">, "Multiplot Representation Out"=w178:T13)  [unwired: 3 in, 3 out]
        n49 = Bundle By Name(cluster=w176, "3D Mesh.lvclass"=w177) -> (w175:T3)
        n50 = event-data() -> ()  [unwired: 1 in, 2 out]
      }
      event Shortcut Menu Selection (User) {
        n51 = event-data() -> ("ItemTag"=w209:string)  [unwired: 1 out]
        n52 = case shown="\"USER_PLOT_PROPERTIES\"" w209 {
          selector: w209 -> [w228 _ _ _ _ _ _]
          tunnel: w211 -> [w225 w274 w310 w317 w324 w345 w371]
          tunnel: [w224 w273 w310 w317 w324 w344 w370] -> w210
          tunnel: w215 -> [w229 w264 w308 w323 w331 w350 w369]
          tunnel: [w229 w271 w307 w323 w331 w350 w369] -> w214
          tunnel: w213 -> [w221 w267 w313 w322 w326 w353 w366]
          tunnel: [w222 w266 w313 w322 w326 w352 w365] -> w212
          tunnel: w203 -> [w218 w259 w314 w321 w330 w343 w368]
          tunnel: [w217 w270 w314 w321 w330 w343 w368] -> w202
          tunnel: w201 -> [w216 w257 w311 w318 w329 w342 w367]
          tunnel: [w216 w268 w311 w318 w329 w342 w367] -> w200
          tunnel: w199 -> [w220 w255 w315 w320 w328 w339 w362]
          tunnel: [w220 w254 w315 w320 w328 w339 w362] -> w198
          tunnel: [w219 w265 w312 w319 w325 w333 w356] -> w197
          tunnel: w196 -> [w219 w265 w312 w319 w325 _ _]
          frame Default {
            n53 = Match Pattern(string=w228, regular expression="ACTIVE_PLOT_") -> (after substring=w223:string, offset past match=w226:i32)  [unwired: 3 out]
            n54 = case shown="Default" w226 {
              tunnel: w225 -> [w240 w250]
              tunnel: [w239 w250] -> w224
              tunnel: w223 -> [w246 _]
              tunnel: [w241 w249] -> w222
              tunnel: w221 -> [w242 w249]
              tunnel: w218 -> [w231 w248]
              tunnel: [w230 w248] -> w217
              frame Default {
                w243 = T17 9 items=["Attribute", "Show/Hide", "Cursor Move", "Zoom", "Mouse Drag", "XY Projection", "YZ Projection", "XZ Projection", "3D Projection", "Active Plot", "Scale"] ("Global String")
                n55 = Decimal String To Number(string=w246) -> (number=w236:i32)  [unwired: 3 out]
                n56 = Unbundle By Name(w240) -> ("3D Mesh.lvclass"=w247:refnum<class "3D Mesh.lvclass">, "Control Ref Queue"=w234:T4)
                n57 = control-ref of="Active Plot"() -> (w238:refnum<vi>)
                n58 = property class="Ring (strict)"(reference=w238, "Value"=w236) -> (error out=w237:errorcluster)  [unwired: 1 in, 1 out]
                n59 = call-dynamic "Write Active Plot.vi"("error in (no error)"=w237, "Active Plot"=w236, "3D Mesh.lvclass in"=w247) -> ("error out"=w232:errorcluster, "3D Mesh.lvclass out"=w233:refnum<class "3D Mesh.lvclass">)  [unwired: 7 in]
                n60 = call <vilib>:"3DMathPlot Action String.vi"("Global String"=w243) -> ("String Out"=w244:string)  [unwired: 10 out]
                n61 = call-dynamic "Graph Color Legend.vi"("Control Ref Queue"=w234, "Multiplot Representation In"=w231, "error in (no error)"=w232, "3D Plot.lvclass in"=w233) -> ("3D Plot.lvclass out"=w235:refnum<class "3D Mesh.lvclass">, "Multiplot Representation Out"=w230:T13)  [unwired: 2 in, 4 out]
                n62 = Bundle By Name(cluster=w242, "State Changed?"=TRUE ("Data Changed?"), "Action Name"=w244) -> (w241:T2)
                n63 = Bundle By Name(cluster=w240, "3D Mesh.lvclass"=w235) -> (w239:T3)
              }
              frame -1 {
              }
            }
          }
          frame "USER_PLOT_PROPERTIES" {
            n64 = Unbundle By Name(w274) -> ("3D Mesh.lvclass"=w272:refnum<class "3D Mesh.lvclass">, "Control Ref Queue"=w251:T4)
            n65 = call-dynamic "Property Dialog.vi"("Control Ref Queue"=w251, "Data"=w255, "Object Cluster In"=w264, "3D Mesh in"=w272) -> ("error out"=w253:errorcluster, "Object Cluster Out"=w262:T16, "3D Mesh out"=w261:refnum<class "3D Mesh.lvclass">, "Cancel?"=w263:bool)  [unwired: 1 in, 3 out]
            n66 = call <vilib>:"Get Scene Data.vi"("Control Ref Queue"=w251, "Multiplot Representation In"=w259, "error in (no error)"=w253, "Data In"=w255, "Actual Transform In"=w257, "3D Plot.lvclass in"=w261) -> ("error out"=w252:errorcluster, "Data Out"=w254:refnum<class "3D Plot Datatype.lvclass">[], "Actual Transform Out"=w256:T11, "3D Plot.lvclass out"=w260:refnum<class "3D Mesh.lvclass">, "Multiplot Representation Out"=w258:T13)  [unwired: 1 out]
            n67 = case shown="False" w263 {
              selector: w263 -> [w276 _]
              tunnel: w262 -> [w284 w299]
              tunnel: w258 -> [w285 w290]
              tunnel: [w284 w306] -> w271
              tunnel: [w285 w293] -> w270
              tunnel: w260 -> [w279 w288]
              tunnel: w252 -> [w278 w289]
              tunnel: [w277 w303] -> w269
              tunnel: [w286 w292] -> w268
              tunnel: w256 -> [w286 w287]
              tunnel: w267 -> [w281 w300]
              tunnel: [w280 w300] -> w266
              tunnel: w251 -> [_ w291]
              frame False {
                w282 = T17 0 items=["Attribute", "Show/Hide", "Cursor Move", "Zoom", "Mouse Drag", "XY Projection", "YZ Projection", "XZ Projection", "3D Projection", "Active Plot", "Scale"] ("Global String")
                n68 = call-dynamic "Backup Plot Name.vi"("error in (no error)"=w278, "3D Mesh.lvclass in"=w279) -> ("3D Mesh.lvclass out"=w277:refnum<class "3D Mesh.lvclass">)  [unwired: 9 out]
                n69 = Not(x=w276) -> (.not. x?=w275:bool)
                n70 = call <vilib>:"3DMathPlot Action String.vi"("Global String"=w282) -> ("String Out"=w283:string)  [unwired: 10 out]
                n71 = Bundle By Name(cluster=w281, "State Changed?"=w275, "Action Name"=w283) -> (w280:T2)
              }
              frame True {
                n72 = call <vilib>:"Scene Settings.vi"("Control Ref Queue"=w291, "error in (no error)"=w289, "Actual Transform In"=w287, "3D Plot.lvclass in"=w288) -> ("error out"=w295:errorcluster, "Actual Transform Out"=w305:T11, "3D Plot.lvclass out"=w296:refnum<class "3D Mesh.lvclass">)  [unwired: 3 in, 2 out]
                n73 = call <vilib>:"Update Scene Object.vi"("Action"=T9 {"Light Action"=enum."Update", "Axis Action"=enum."Update", "Plot Action"=enum."Update", "Cursor Action"=enum."Update", "Fast Draw Action"=enum."Nothing"}, "Control Ref Queue"=w291, "Multiplot Representation In"=w290, "error in (no error)"=w295, "Object Cluster In"=w299, "Actual Transform In"=w305, "3D Plot.lvclass in"=w296) -> ("error out"=w302:errorcluster, "Object Cluster Out"=w306:T16, "Actual Transform Out"=w292:T11, "3D Plot.lvclass out"=w304:refnum<class "3D Mesh.lvclass">, "Multiplot Representation Out"=w294:T13)
                n74 = call-dynamic "Graph Color Legend.vi"("Control Ref Queue"=w291, "Multiplot Representation In"=w294, "error in (no error)"=w302, "3D Plot.lvclass in"=w304) -> ("error out"=w298:errorcluster, "3D Plot.lvclass out"=w303:refnum<class "3D Mesh.lvclass">, "Multiplot Representation Out"=w293:T13)  [unwired: 2 in, 3 out]
                n75 = invoke on="3D Picture Control" class="SceneGraphDisp (strict)" method="Redraw"(error in=w298) -> (error out=w297:errorcluster)  [unwired: 2 in, 2 out]
                n76 = call <vilib>:"Render Window Redraw.vi"("Control Ref Queue"=w291, "error in (no error)"=w297) -> ()  [unwired: 1 in, 9 out]
              }
            }
            n77 = Bundle By Name(cluster=w274, "3D Mesh.lvclass"=w269) -> (w273:T3)
          }
          frame "USER_RENDER_WINDOW" {
            n78 = Unbundle By Name(w310) -> ("Control Ref Queue"=w309:T4)
            n79 = call <vilib>:"Render Window Open.vi"("Control Ref Queue"=w309, "Object Cluster In"=w308) -> ("Object Cluster Out"=w307:T16)  [unwired: 3 in, 6 out]
          }
          frame "USER_EXPORT_IMAGE" {
            n80 = Unbundle By Name(w317) -> ("Control Ref Queue"=w316:T4)
            n81 = call <vilib>:"Image File Dialog.vi"("Control Ref Queue"=w316) -> ()  [unwired: 2 in, 9 out]
          }
          frame "USER_PRINT_IMAGE" {
            n82 = Unbundle By Name(w324) -> ("Control Ref Queue"=w327:T4)
            n83 = call <vilib>:"Image to Printer.vi"("Control Ref Queue"=w327) -> ()  [unwired: 1 in, 10 out]
          }
          frame "USER_PROJECTION_VISIBLE" {
            w341 = T17 1 items=["Attribute", "Show/Hide", "Cursor Move", "Zoom", "Mouse Drag", "XY Projection", "YZ Projection", "XZ Projection", "3D Projection", "Active Plot", "Scale"] ("Global String")
            n84 = Unbundle By Name(w345) -> ("3D Mesh.lvclass"=w349:refnum<class "3D Mesh.lvclass">, "Control Ref Queue"=w332:T4)
            n85 = call <vilib>:"Read Property.vi"("3D Plot.lvclass in"=w349) -> ("error out"=w334:errorcluster, "Property Cluster"=w347:T18, "3D Plot.lvclass out"=w348:refnum<class "3D Mesh.lvclass">)  [unwired: 1 in, 7 out]
            n86 = Unbundle By Name(w347) -> ("Appearance Property.Visibility.Projection Palette"=w351:bool)
            n87 = Not(x=w351) -> (.not. x?=w338:bool)
            n88 = Bundle By Name(cluster=w347, "Appearance Property.Visibility.Projection Palette"=w338) -> (w346:T18)
            n89 = call <vilib>:"3DMathPlot Action String.vi"("Global String"=w341) -> ("String Out"=w340:string)  [unwired: 10 out]
            n90 = call <vilib>:"Write Property.vi"("error in (no error)"=w334, "Property Cluster"=w346, "3D Plot.lvclass in"=w348) -> ("error out"=w337:errorcluster, "3D Plot.lvclass out"=w336:refnum<class "3D Mesh.lvclass">)  [unwired: 7 out]
            n91 = Bundle By Name(cluster=w353, "State Changed?"=TRUE ("Data Changed?"), "Action Name"=w340) -> (w352:T2)
            n92 = call <vilib>:"Update Palette with Ramp.vi"("Control Ref Queue"=w332, "error in (no error)"=w337, "3D Plot.lvclass in"=w336) -> ("Ignore the size change?"=w333:bool, "3D Plot.lvclass out"=w335:refnum<class "3D Mesh.lvclass">)  [unwired: 7 out]
            n93 = Bundle By Name(cluster=w345, "3D Mesh.lvclass"=w335) -> (w344:T3)
          }
          frame "USER_COLOR_RAMP_VISIBLE" {
            w363 = T17 1 items=["Attribute", "Show/Hide", "Cursor Move", "Zoom", "Mouse Drag", "XY Projection", "YZ Projection", "XZ Projection", "3D Projection", "Active Plot", "Scale"] ("Global String")
            n94 = Unbundle By Name(w371) -> ("3D Mesh.lvclass"=w375:refnum<class "3D Mesh.lvclass">, "Control Ref Queue"=w355:T4)
            n95 = call <vilib>:"Read Property.vi"("3D Plot.lvclass in"=w375) -> ("error out"=w357:errorcluster, "Property Cluster"=w374:T18, "3D Plot.lvclass out"=w361:refnum<class "3D Mesh.lvclass">)  [unwired: 1 in, 7 out]
            n96 = Unbundle By Name(w374) -> ("Appearance Property.Visibility.Color Ramp Palette"=w376:bool)
            n97 = Not(x=w376) -> (.not. x?=w364:bool)
            n98 = Bundle By Name(cluster=w374, "Appearance Property.Visibility.Color Ramp Palette"=w364) -> (w373:T18)
            n99 = call <vilib>:"3DMathPlot Action String.vi"("Global String"=w363) -> ("String Out"=w372:string)  [unwired: 10 out]
            n100 = call <vilib>:"Write Property.vi"("error in (no error)"=w357, "Property Cluster"=w373, "3D Plot.lvclass in"=w361) -> ("error out"=w360:errorcluster, "3D Plot.lvclass out"=w359:refnum<class "3D Mesh.lvclass">)  [unwired: 7 out]
            n101 = Bundle By Name(cluster=w366, "State Changed?"=TRUE ("Data Changed?"), "Action Name"=w372) -> (w365:T2)
            n102 = call <vilib>:"Update Palette with Ramp.vi"("Control Ref Queue"=w355, "error in (no error)"=w360, "3D Plot.lvclass in"=w359) -> ("Ignore the size change?"=w356:bool, "3D Plot.lvclass out"=w358:refnum<class "3D Mesh.lvclass">)  [unwired: 7 out]
            n103 = Bundle By Name(cluster=w371, "3D Mesh.lvclass"=w358) -> (w370:T3)
          }
        }
      }
      event "3D Picture Control": Mouse Down {
        n104 = event-data() -> ("PlatMods.Shift"=w400:bool, "Button"=w380:u16, "PlatMods.Ctrl"=w378:bool)  [unwired: 1 out]
        n105 = call <vilib>:"Check Right Click.vi"("Ctrl"=w378, "Button"=w380) -> ("Right Click?"=w379:bool)  [unwired: 9 out]
        n106 = case shown="False" w379 {
          tunnel: w400 -> [_ w431]
          tunnel: w399 -> [w410 w428]
          tunnel: w398 -> [_ w430]
          tunnel: [w410 w411] -> w381
          tunnel: [w409 w426] -> w397
          tunnel: w396 -> [w409 w425]
          tunnel: w394 -> [w408 w424]
          tunnel: [w408 w423] -> w393
          tunnel: w392 -> [w407 w421]
          tunnel: [w407 w421] -> w391
          tunnel: [w406 w422] -> w390
          tunnel: w389 -> [w406 w420]
          tunnel: [w405 w419] -> w387
          tunnel: w386 -> [w405 w418]
          tunnel: w385 -> [w403 w415]
          tunnel: w384 -> [w404 w414]
          tunnel: [w404 w413] -> w383
          tunnel: [w403 w412] -> w382
          frame True {
          }
          frame False {
            n107 = Unbundle By Name(w430) -> ("3D Mesh.lvclass"=w429:refnum<class "3D Mesh.lvclass">, "Control Ref Queue"=w417:T4)
            n108 = call <vilib>:"Read Property.vi"("3D Plot.lvclass in"=w429) -> ("Property Cluster"=w427:T18, "3D Plot.lvclass out"=w416:refnum<class "3D Mesh.lvclass">)  [unwired: 1 in, 8 out]
            n109 = case shown="False" w421 {
              selector: w421 -> [_ w467]
              tunnel: w431 -> [w441 _]
              tunnel: w427 -> [w444 w470]
              tunnel: w428 -> [w449 w463]
              tunnel: [w441 w468] -> w426
              tunnel: w425 -> [_ w468]
              tunnel: w424 -> [w443 _]
              tunnel: [w443 w467] -> w423
              tunnel: [w442 w469] -> w422
              tunnel: w420 -> [w442 _]
              tunnel: [w440 w466] -> w419
              tunnel: w418 -> [_ w466]
              tunnel: w417 -> [w438 _]
              tunnel: w416 -> [w437 _]
              tunnel: w415 -> [w436 w464]
              tunnel: w414 -> [w435 w465]
              tunnel: [w434 w465] -> w413
              tunnel: [w433 w464] -> w412
              tunnel: [w432 w463] -> w411
              frame False {
                n110 = Unbundle By Name(w444) -> ("Graph Property.General Property.Fast Draw?"=w447:bool, "Graph Property.View Property.View Direction"=w448:T10, "Graph Property.View Property.User Defined View Direction.View Distance"=w440:sgl)
                n111 = Equal?(x=w448, y=T10."User Defined") -> (x = y?=w446:bool)
                n112 = And(x=w447, y=w446) -> (x .and. y?=w445:bool)
                n113 = case shown="True" w445 {
                  tunnel: w449 -> [w450 w461]
                  tunnel: w438 -> [_ w460]
                  tunnel: w437 -> [_ w459]
                  tunnel: w436 -> [w451 w458]
                  tunnel: w435 -> [w452 w457]
                  tunnel: [w452 w455] -> w434
                  tunnel: [w451 w454] -> w433
                  tunnel: [w450 w453] -> w432
                  frame False {
                  }
                  frame True {
                    # "Update the Fast Draw and display it."
                    n114 = call <vilib>:"Update Scene Object.vi"("Action"=T9 {"Light Action"=enum."Nothing", "Axis Action"=enum."Nothing", "Plot Action"=enum."Nothing", "Cursor Action"=enum."Nothing", "Fast Draw Action"=enum."Update"}, "Control Ref Queue"=w460, "Multiplot Representation In"=w457, "Object Cluster In"=w461, "Actual Transform In"=w458, "3D Plot.lvclass in"=w459) -> ("Object Cluster Out"=w453:T16, "Actual Transform Out"=w454:T11, "Multiplot Representation Out"=w455:T13)  [unwired: 1 in, 2 out]
                    n115 = Unbundle By Name(w453) -> ("Fast Root Scene Object"=w462:refnum<vi>)
                    n116 = local write "3D Picture Control"(w462) -> ()
                  }
                }
              }
              frame True {
                n117 = Unbundle By Name(w470) -> ("Cursor Property Array"=w469:T34)
              }
            }
          }
        }
      }
      event "3D Picture Control": Mouse Up {
        w477 = FALSE
        n118 = event-data() -> ("Button"=w482:u16)  [unwired: 1 out]
        n119 = case shown="1" w482 {
          tunnel: w485 -> [w493 w528]
          tunnel: w488 -> [w494 w510]
          tunnel: [w492 w518] -> w483
          tunnel: [w494 w515] -> w487
          tunnel: [w493 w527] -> w484
          tunnel: w481 -> [_ w525]
          tunnel: w480 -> [_ w524]
          tunnel: w479 -> [_ w520]
          tunnel: w486 -> [w492 w519]
          tunnel: w476 -> [w491 w504]
          tunnel: [w491 w505] -> w475
          tunnel: w474 -> [w490 w508]
          tunnel: [w490 w506] -> w473
          tunnel: w471 -> [_ w513]
          frame 0, Default {
          }
          frame 1 {
            n120 = Build Array(w525, w524) -> (w523:bool[])
            n121 = Unbundle By Name(w519) -> ("3D Mesh.lvclass"=w502:refnum<class "3D Mesh.lvclass">, "Control Ref Queue"=w509:T4)
            n122 = Boolean Array To Number(Boolean array=w523) -> (number=w522:u32)
            n123 = call <vilib>:"Read Property.vi"("3D Plot.lvclass in"=w502) -> ("error out"=w496:errorcluster, "Property Cluster"=w499:T18, "3D Plot.lvclass out"=w503:refnum<class "3D Mesh.lvclass">)  [unwired: 1 in, 7 out]
            n124 = case shown="0, Default" w522 {
              tunnel: [w536 w542 w547] -> w526
              tunnel: [w531 TRUE ("State Changed?") TRUE ("State Changed?")] -> w521
              tunnel: w520 -> [_ _ w549]
              tunnel: w509 -> [w534 _ _]
              tunnel: w513 -> [_ w540 _]
              tunnel: w499 -> [w533 w539 w546]
              tunnel: [w532 w538 w545] -> w498
              tunnel: w496 -> [w530 w537 w544]
              tunnel: [w529 w537 w544] -> w495
              frame 0, Default {
                w535 = T17 4 items=["Attribute", "Show/Hide", "Cursor Move", "Zoom", "Mouse Drag", "XY Projection", "YZ Projection", "XZ Projection", "3D Projection", "Active Plot", "Scale"] ("Global String")
                n125 = call <vilib>:"Get Latitude & Longitude.vi"("Control Ref Queue"=w534, "error in (no error)"=w530, "Property Cluster in"=w533) -> ("error out"=w529:errorcluster, "State Changed?"=w531:bool, "Property Cluster out"=w532:T18)  [unwired: 6 out]
                n126 = call <vilib>:"3DMathPlot Action String.vi"("Global String"=w535) -> ("String Out"=w536:string)  [unwired: 10 out]
              }
              frame 1 {
                w541 = T17 3 items=["Attribute", "Show/Hide", "Cursor Move", "Zoom", "Mouse Drag", "XY Projection", "YZ Projection", "XZ Projection", "3D Projection", "Active Plot", "Scale"] ("Global String")
                n127 = Bundle By Name(cluster=w539, "Graph Property.View Property.User Defined View Direction.View Distance"=w540) -> (w538:T18)
                n128 = call <vilib>:"3DMathPlot Action String.vi"("Global String"=w541) -> ("String Out"=w542:string)  [unwired: 10 out]
              }
              frame 2 {
                w548 = T17 2 items=["Attribute", "Show/Hide", "Cursor Move", "Zoom", "Mouse Drag", "XY Projection", "YZ Projection", "XZ Projection", "3D Projection", "Active Plot", "Scale"] ("Global String")
                n129 = Bundle By Name(cluster=w546, "Cursor Property Array"=w549) -> (w545:T18)
                n130 = call <vilib>:"3DMathPlot Action String.vi"("Global String"=w548) -> ("String Out"=w547:string)  [unwired: 10 out]
              }
            }
            n131 = call <vilib>:"Write Property.vi"("error in (no error)"=w495, "Property Cluster"=w498, "3D Plot.lvclass in"=w503) -> ("error out"=w500:errorcluster, "3D Plot.lvclass out"=w501:refnum<class "3D Mesh.lvclass">)  [unwired: 7 out]
            n132 = call <vilib>:"Scene Settings.vi"("Control Ref Queue"=w509, "error in (no error)"=w500, "Actual Transform In"=w508, "3D Plot.lvclass in"=w501) -> ("error out"=w512:errorcluster, "Actual Transform Out"=w507:T11, "3D Plot.lvclass out"=w511:refnum<class "3D Mesh.lvclass">)  [unwired: 3 in, 2 out]
            n133 = call <vilib>:"Update Scene Object.vi"("Action"=T9 {"Light Action"=enum."Nothing", "Axis Action"=enum."Nothing", "Plot Action"=enum."Nothing", "Cursor Action"=enum."Update", "Fast Draw Action"=enum."Nothing"}, "Control Ref Queue"=w509, "Multiplot Representation In"=w504, "error in (no error)"=w512, "Object Cluster In"=w510, "Actual Transform In"=w507, "3D Plot.lvclass in"=w511) -> ("error out"=w514:errorcluster, "Object Cluster Out"=w515:T16, "Actual Transform Out"=w506:T11, "3D Plot.lvclass out"=w497:refnum<class "3D Mesh.lvclass">, "Multiplot Representation Out"=w505:T13)
            n134 = Unbundle By Name(w515) -> ("Root Scene Object"=w516:refnum<vi>)
            n135 = call <vilib>:"Render Window Redraw.vi"("Control Ref Queue"=w509, "error in (no error)"=w514) -> ()  [unwired: 1 in, 9 out]
            n136 = Bundle By Name(cluster=w528, "State Changed?"=w521, "Action Name"=w526) -> (w527:T2)
            n137 = local write "3D Picture Control"(w516) -> ()
            n138 = Bundle By Name(cluster=w519, "3D Mesh.lvclass"=w497) -> (w518:T3)
          }
        }
      }
      event "3D Picture Control": Mouse Move {
        n139 = event-data() -> ("Coords"=w554:T45)  [unwired: 1 out]
        n140 = Unbundle By Name(w569) -> ("3D Mesh.lvclass"=w553:refnum<class "3D Mesh.lvclass">, "Control Ref Queue"=w556:T4)
        n141 = call <vilib>:"Plot Zoom.vi"("Control Ref Queue"=w556, "Zoom Mode"=w571, "3D Plot.lvclass in"=w553) -> ("error out"=w568:errorcluster, "Dup Ortho Zoom Mode"=w570:bool, "3D Plot.lvclass out"=w552:refnum<class "3D Mesh.lvclass">, "View Distance Out"=w551:sgl)  [unwired: 2 in, 3 out]
        n142 = call <vilib>:"Cursor Move.vi"("3D Plot.lvclass in"=w552, "Coords"=w554, "Control Ref Queue"=w556, "Actual Transform In"=w558, "Object Cluster In"=w567, "Cursor ID In"=w565, "Tracking Cursor?"=w561, "error in (no error)"=w568, "Multiplot Represention"=w559) -> ("Object Cluster Out"=w566:T16, "Cursor ID"=w564:i32, "Drag Cursor?"=w560:bool, "Update Plot?"=w562:bool, "Cursor Property Array"=w563:T34, "error out"=w555:errorcluster)  [unwired: 1 out]
        n143 = case shown="True" w562 {
          tunnel: w555 -> [_ w574]
          frame False {
          }
          frame True {
            n144 = invoke on="3D Picture Control" class="SceneGraphDisp (strict)" method="Redraw"(error in=w574) -> ()  [unwired: 2 in, 3 out]
          }
        }
      }
      event "Projection Palette.XY Projection": Value Change {
        w590 = T17 5 items=["Attribute", "Show/Hide", "Cursor Move", "Zoom", "Mouse Drag", "XY Projection", "YZ Projection", "XZ Projection", "3D Projection", "Active Plot", "Scale"] ("Global String")
        n145 = event-data() -> ("NewVal"=w576:bool)  [unwired: 1 out]
        n146 = Unbundle By Name(w595) -> ("3D Mesh.lvclass"=w582:refnum<class "3D Mesh.lvclass">, "Control Ref Queue"=w575:T4)
        n147 = call <vilib>:"View Direction Write.vi"("Control Ref Queue"=w575, "View Direction"=T10."Towards X-Y Plane", "3D Plot.lvclass in"=w582) -> ("error out"=w580:errorcluster, "3D Plot.lvclass out"=w581:refnum<class "3D Mesh.lvclass">)  [unwired: 1 in, 6 out]
        n148 = call <vilib>:"Scene Settings.vi"("Control Ref Queue"=w575, "error in (no error)"=w580, "Actual Transform In"=w579, "3D Plot.lvclass in"=w581) -> ("error out"=w584:errorcluster, "Actual Transform Out"=w578:T11, "3D Plot.lvclass out"=w586:refnum<class "3D Mesh.lvclass">)  [unwired: 3 in, 2 out]
        n149 = call <vilib>:"3DMathPlot Action String.vi"("Global String"=w590) -> ("String Out"=w591:string)  [unwired: 10 out]
        n150 = invoke on="3D Picture Control" class="SceneGraphDisp (strict)" method="Redraw"(error in=w584) -> (error out=w588:errorcluster)  [unwired: 2 in, 2 out]
        n151 = Bundle By Name(cluster=w594, "State Changed?"=w576, "Action Name"=w591) -> (w593:T2)
        n152 = call <vilib>:"Render Window Redraw.vi"("Control Ref Queue"=w575, "error in (no error)"=w588) -> ()  [unwired: 1 in, 9 out]
        n153 = Bundle By Name(cluster=w595, "3D Mesh.lvclass"=w586) -> (w592:T3)
      }
      event "Projection Palette.XZ Projection": Value Change {
        w617 = T17 7 items=["Attribute", "Show/Hide", "Cursor Move", "Zoom", "Mouse Drag", "XY Projection", "YZ Projection", "XZ Projection", "3D Projection", "Active Plot", "Scale"] ("Global String")
        n154 = event-data() -> ("NewVal"=w603:bool)  [unwired: 1 out]
        n155 = Unbundle By Name(w622) -> ("3D Mesh.lvclass"=w607:refnum<class "3D Mesh.lvclass">, "Control Ref Queue"=w602:T4)
        n156 = call <vilib>:"View Direction Write.vi"("Control Ref Queue"=w602, "View Direction"=T10."Towards X-Z Plane", "3D Plot.lvclass in"=w607) -> ("error out"=w605:errorcluster, "3D Plot.lvclass out"=w606:refnum<class "3D Mesh.lvclass">)  [unwired: 1 in, 6 out]
        n157 = call <vilib>:"Scene Settings.vi"("Control Ref Queue"=w602, "error in (no error)"=w605, "Actual Transform In"=w609, "3D Plot.lvclass in"=w606) -> ("error out"=w611:errorcluster, "Actual Transform Out"=w608:T11, "3D Plot.lvclass out"=w612:refnum<class "3D Mesh.lvclass">)  [unwired: 4 in, 1 out]
        n158 = call <vilib>:"3DMathPlot Action String.vi"("Global String"=w617) -> ("String Out"=w618:string)  [unwired: 10 out]
        n159 = invoke on="3D Picture Control" class="SceneGraphDisp (strict)" method="Redraw"(error in=w611) -> (error out=w615:errorcluster)  [unwired: 2 in, 2 out]
        n160 = Bundle By Name(cluster=w620, "State Changed?"=w603, "Action Name"=w618) -> (w619:T2)
        n161 = call <vilib>:"Render Window Redraw.vi"("Control Ref Queue"=w602, "error in (no error)"=w615) -> ()  [unwired: 1 in, 9 out]
        n162 = Bundle By Name(cluster=w622, "3D Mesh.lvclass"=w612) -> (w621:T3)
      }
      event "Projection Palette.YZ Projection": Value Change {
        w644 = T17 6 items=["Attribute", "Show/Hide", "Cursor Move", "Zoom", "Mouse Drag", "XY Projection", "YZ Projection", "XZ Projection", "3D Projection", "Active Plot", "Scale"] ("Global String")
        n163 = event-data() -> ("NewVal"=w630:bool)  [unwired: 1 out]
        n164 = Unbundle By Name(w649) -> ("3D Mesh.lvclass"=w634:refnum<class "3D Mesh.lvclass">, "Control Ref Queue"=w629:T4)
        n165 = call <vilib>:"View Direction Write.vi"("Control Ref Queue"=w629, "View Direction"=T10."Towards Y-Z Plane", "3D Plot.lvclass in"=w634) -> ("error out"=w632:errorcluster, "3D Plot.lvclass out"=w633:refnum<class "3D Mesh.lvclass">)  [unwired: 1 in, 6 out]
        n166 = call <vilib>:"Scene Settings.vi"("Control Ref Queue"=w629, "error in (no error)"=w632, "Actual Transform In"=w636, "3D Plot.lvclass in"=w633) -> ("error out"=w638:errorcluster, "Actual Transform Out"=w635:T11, "3D Plot.lvclass out"=w640:refnum<class "3D Mesh.lvclass">)  [unwired: 3 in, 2 out]
        n167 = call <vilib>:"3DMathPlot Action String.vi"("Global String"=w644) -> ("String Out"=w645:string)  [unwired: 10 out]
        n168 = invoke on="3D Picture Control" class="SceneGraphDisp (strict)" method="Redraw"(error in=w638) -> (error out=w642:errorcluster)  [unwired: 2 in, 2 out]
        n169 = Bundle By Name(cluster=w647, "State Changed?"=w630, "Action Name"=w645) -> (w646:T2)
        n170 = call <vilib>:"Render Window Redraw.vi"("Control Ref Queue"=w629, "error in (no error)"=w642) -> ()  [unwired: 1 in, 9 out]
        n171 = Bundle By Name(cluster=w649, "3D Mesh.lvclass"=w640) -> (w648:T3)
      }
      event "Projection Palette.3D Projection": Value Change {
        w671 = T17 8 items=["Attribute", "Show/Hide", "Cursor Move", "Zoom", "Mouse Drag", "XY Projection", "YZ Projection", "XZ Projection", "3D Projection", "Active Plot", "Scale"] ("Global String")
        n172 = event-data() -> ("NewVal"=w657:bool)  [unwired: 1 out]
        n173 = Unbundle By Name(w676) -> ("3D Mesh.lvclass"=w661:refnum<class "3D Mesh.lvclass">, "Control Ref Queue"=w656:T4)
        n174 = call <vilib>:"View Direction Write.vi"("Control Ref Queue"=w656, "View Direction"=T10."User Defined", "3D Plot.lvclass in"=w661) -> ("error out"=w659:errorcluster, "3D Plot.lvclass out"=w660:refnum<class "3D Mesh.lvclass">)  [unwired: 1 in, 6 out]
        n175 = call <vilib>:"Scene Settings.vi"("Control Ref Queue"=w656, "error in (no error)"=w659, "Actual Transform In"=w663, "3D Plot.lvclass in"=w660) -> ("error out"=w666:errorcluster, "Actual Transform Out"=w662:T11, "3D Plot.lvclass out"=w665:refnum<class "3D Mesh.lvclass">)  [unwired: 3 in, 2 out]
        n176 = call <vilib>:"3DMathPlot Action String.vi"("Global String"=w671) -> ("String Out"=w672:string)  [unwired: 10 out]
        n177 = invoke on="3D Picture Control" class="SceneGraphDisp (strict)" method="Redraw"(error in=w666) -> (error out=w669:errorcluster)  [unwired: 2 in, 2 out]
        n178 = Bundle By Name(cluster=w674, "State Changed?"=w657, "Action Name"=w672) -> (w673:T2)
        n179 = call <vilib>:"Render Window Redraw.vi"("Control Ref Queue"=w656, "error in (no error)"=w669) -> ()  [unwired: 1 in, 9 out]
        n180 = Bundle By Name(cluster=w676, "3D Mesh.lvclass"=w665) -> (w675:T3)
      }
      event "Color Ramp Palette.Active Plot": Value Change {
        w695 = T17 9 items=["Attribute", "Show/Hide", "Cursor Move", "Zoom", "Mouse Drag", "XY Projection", "YZ Projection", "XZ Projection", "3D Projection", "Active Plot", "Scale"] ("Global String")
        n181 = event-data() -> ("NewVal"=w698:i32)  [unwired: 1 out]
        n182 = Unbundle By Name(w700) -> ("3D Mesh.lvclass"=w701:refnum<class "3D Mesh.lvclass">, "Control Ref Queue"=w690:T4)
        n183 = call-dynamic "Write Active Plot.vi"("Active Plot"=w698, "3D Mesh.lvclass in"=w701) -> ("error out"=w685:errorcluster, "3D Mesh.lvclass out"=w686:refnum<class "3D Mesh.lvclass">)  [unwired: 8 in]
        n184 = call <vilib>:"3DMathPlot Action String.vi"("Global String"=w695) -> ("String Out"=w696:string)  [unwired: 10 out]
        n185 = Bundle By Name(cluster=w694, "State Changed?"=TRUE ("Data Changed?"), "Action Name"=w696) -> (w693:T2)
        n186 = call-dynamic "Graph Color Legend.vi"("Control Ref Queue"=w690, "Multiplot Representation In"=w684, "error in (no error)"=w685, "3D Plot.lvclass in"=w686) -> ("3D Plot.lvclass out"=w692:refnum<class "3D Mesh.lvclass">, "Multiplot Representation Out"=w683:T13)  [unwired: 2 in, 4 out]
        n187 = Bundle By Name(cluster=w700, "3D Mesh.lvclass"=w692) -> (w699:T3)
      }
      event "XY Graph": Scale Range Change {
        w723 = T17 10 items=["Attribute", "Show/Hide", "Cursor Move", "Zoom", "Mouse Drag", "XY Projection", "YZ Projection", "XZ Projection", "3D Projection", "Active Plot", "Scale"] ("Global String")
        n188 = event-data() -> ("NewRange"=w734:T46, "Kind"=w733:enum16{"X-Scale", "Y-Scale", "Z-Scale"})  [unwired: 1 out]
        n189 = Unbundle By Name(w731) -> ("3D Mesh.lvclass"=w732:refnum<class "3D Mesh.lvclass">, "Control Ref Queue"=w716:T4)
        n190 = call <vilib>:"Transform Cluster Update.vi"("Axis"=w733, "NewRange"=w734, "Multiplot Representation In"=w709, "Actual Transform In"=w712, "3D Plot in"=w732) -> ("error out"=w718:errorcluster, "Actual Transform Out"=w711:T11, "3D Plot out"=w719:refnum<class "3D Mesh.lvclass">, "Multiplot Representation Out"=w710:T13)  [unwired: 1 in, 2 out]
        n191 = call <vilib>:"Update Scene Object.vi"("Action"=T9 {"Light Action"=enum."Nothing", "Axis Action"=enum."Update", "Plot Action"=enum."Update", "Cursor Action"=enum."Update", "Fast Draw Action"=enum."Nothing"}, "Control Ref Queue"=w716, "Multiplot Representation In"=w710, "error in (no error)"=w718, "Object Cluster In"=w725, "Actual Transform In"=w711, "3D Plot.lvclass in"=w719) -> ("error out"=w720:errorcluster, "Object Cluster Out"=w726:T16, "Actual Transform Out"=w714:T11, "3D Plot.lvclass out"=w708:refnum<class "3D Mesh.lvclass">, "Multiplot Representation Out"=w713:T13)
        n192 = invoke on="3D Picture Control" class="SceneGraphDisp (strict)" method="Redraw"(error in=w720) -> (error out=w717:errorcluster)  [unwired: 2 in, 2 out]
        n193 = call <vilib>:"3DMathPlot Action String.vi"("Global String"=w723) -> ("String Out"=w724:string)  [unwired: 10 out]
        n194 = call <vilib>:"Render Window Redraw.vi"("Control Ref Queue"=w716, "error in (no error)"=w717) -> ()  [unwired: 1 in, 9 out]
        n195 = Bundle By Name(cluster=w728, "State Changed?"=TRUE ("Data Changed?"), "Action Name"=w724) -> (w727:T2)
        n196 = Bundle By Name(cluster=w731, "3D Mesh.lvclass"=w708) -> (w730:T3)
      }
      event Panel Resize {
        n197 = event-data() -> ()  [unwired: 2 out]
        n198 = case shown="False" w745 {
          tunnel: w747 -> [w760 w762]
          tunnel: [w759 w762] -> w746
          frame False {
            n199 = Unbundle By Name(w760) -> ("3D Mesh.lvclass"=w761:refnum<class "3D Mesh.lvclass">, "Control Ref Queue"=w758:T4)
            n200 = call <vilib>:"Panel Resize.vi"("Control Ref Queue"=w758, "3D Plot.lvclass"=w761) -> ("error out"=w756:errorcluster, "3D Plot.lvclass out"=w757:refnum<class "3D Mesh.lvclass">)  [unwired: 3 in, 5 out]
            n201 = invoke on="3D Picture Control" class="SceneGraphDisp (strict)" method="Redraw"(error in=w756) -> ()  [unwired: 2 in, 3 out]
            n202 = Bundle By Name(cluster=w760, "3D Mesh.lvclass"=w757) -> (w759:T3)
          }
          frame True {
          }
        }
      }
    }
  }
  "Display State Out" <- w7
  "Data Out" <- w9
  "Action" <- w6
